vi "REWORK_MAIN.vi"() -> ()   [LabVIEW 2019]
uses:
  REWORK/MAIN/REWORK_station.ctl
  REWORK/MAIN/REWORK_header_data_display.ctl
  REWORK/ini/typedef/REWORK_all_config_info.ctl
  REWORK/ini/typedef/REWORK_main_ini_file.ctl
  REWORK/queues/typedef/REWORK_queue_refnums.ctl
  REWORK/queues/typedef/REWORK_MAIN_queue_element.ctl
  REWORK/MAIN/REWORK_MAIN_sequence_state.ctl
  REWORK/queues/typedef/REWORK_SCANNER_queue_element.ctl
  REWORK/SCANNER/REWORK_SCANNER_sequence_state.ctl
  REWORK/FGV/error_buffer/FGV_REWORK_error_buffer.ctl
  REWORK/TCP/REWORK_TCP_sequence_state.ctl
  REWORK/FGV/connection_reference/FGV_REWORK_connection_reference.ctl
  REWORK/FGV/DIAGNOSTICS_records_display/FGV_REWORK_DIAGNOSTICS_records_display.ctl
  REWORK/FGV/connection_indicators/FGV_REWORK_connection_indicators.ctl
  REWORK/FGV/DIAGNOSTICS_message_history_buffer/FGV_REWORK_DIAGNOSTICS_message_history_buffer.ctl
  REWORK/FGV/SQL_connection/FGV_REWORK_SQL_connection.ctl
  REWORK/FGV/login/FGV_REWORK_login.ctl
  REWORK/FGV/login/REWORK_login_refnums.ctl
  REWORK/FGV/REWORK_records_display/FGV_REWORK_records_display.ctl
  REWORK/FGV/REWORK_records_display/REWORK_references.ctl
  REWORK/FGV/REWORK_status_display/FGV_REWORK_status_display.ctl
  REWORK/FGV/REWORK_destination_selector/FGV_REWORK_destination_selector.ctl
  _misc/PLC_connection_status.ctl
  REWORK/MAIN/REWORK_thread.ctl
  <vilib>/Utility/miscctls.llb/LVRowAndColumnTypeDef.ctl
  _misc/AULocalize/SubVIs/RegisterVI.vi
  _misc/byte_array_parser/to_string.vi
  <vilib>/Instr/_visa.llb/VISA Configure Serial Port (Instr).vi
panel:
  out "app_title":string caption="A603 - Rework"
  in  "REWORK_toggle_all_results":bool
  in  "USER_login_logout":bool
  out "SQL_connections_indicator_global":bool=TRUE caption="SQL Connection Status:"
  out "PLC_connections_indicator_global":bool=TRUE caption="PLC Connection Status:"
  in  "STOP":bool
  out "ERROR_indicator_global":bool caption="Application Status:"
  out "current_access_level":i32=10 caption="Access level:"
  out "current_username":string="jlonga" caption="Logged in as:"
  in  "main_tab":enum32{"Rework", "Diagnostics", "Errors"}(tab)
  out "input_header":string caption="INPUT"
  in  "REWORK_clear_gear_data":bool
  in  "REWORK_read_data":bool
  in  "REWORK_destination":u16(ring) caption="Rework:" items=["NO REWORK POSSIBLE FOR THIS GEAR"]
  in  "REWORK_toggle_all_results":bool
  in  "REWORK_commit":bool
  in  "REWORK_records":i32(listbox)=-1
  out "REWORK_status":string
  in  "REWORK_gear_serial":string caption="Gear Serial:"
  in  "REWORK_station_filter":T1 caption="Station:" items=["ALL"=0, "Station 10"=10, "Station 20"=20, "Station 30"=30, "Station 40"=40, "Station 50"=50, "Station 60"=60, "Station 70"=70, "Station 80"=80, "Station 90"=90, "Station 100"=100, "Station 110"=110, "Station 120"=120, "Station 160"=165]
  out "REWORK_header_data_display":T2
  out "gear_info_summary_header":string caption="GEAR INFO SUMMARY"
  out "gear_serial_display":string
  in  "DIAGNOSTICS_save_log":bool
  in  "DIAGNOSTICS_show_messages":bool
  in  "DIAGNOSTICS_records":i32(listbox)
  in  "ERROR_records":i32(listbox)
  in  "ERROR_clear":bool
  out "ERROR_indicator_tab":bool
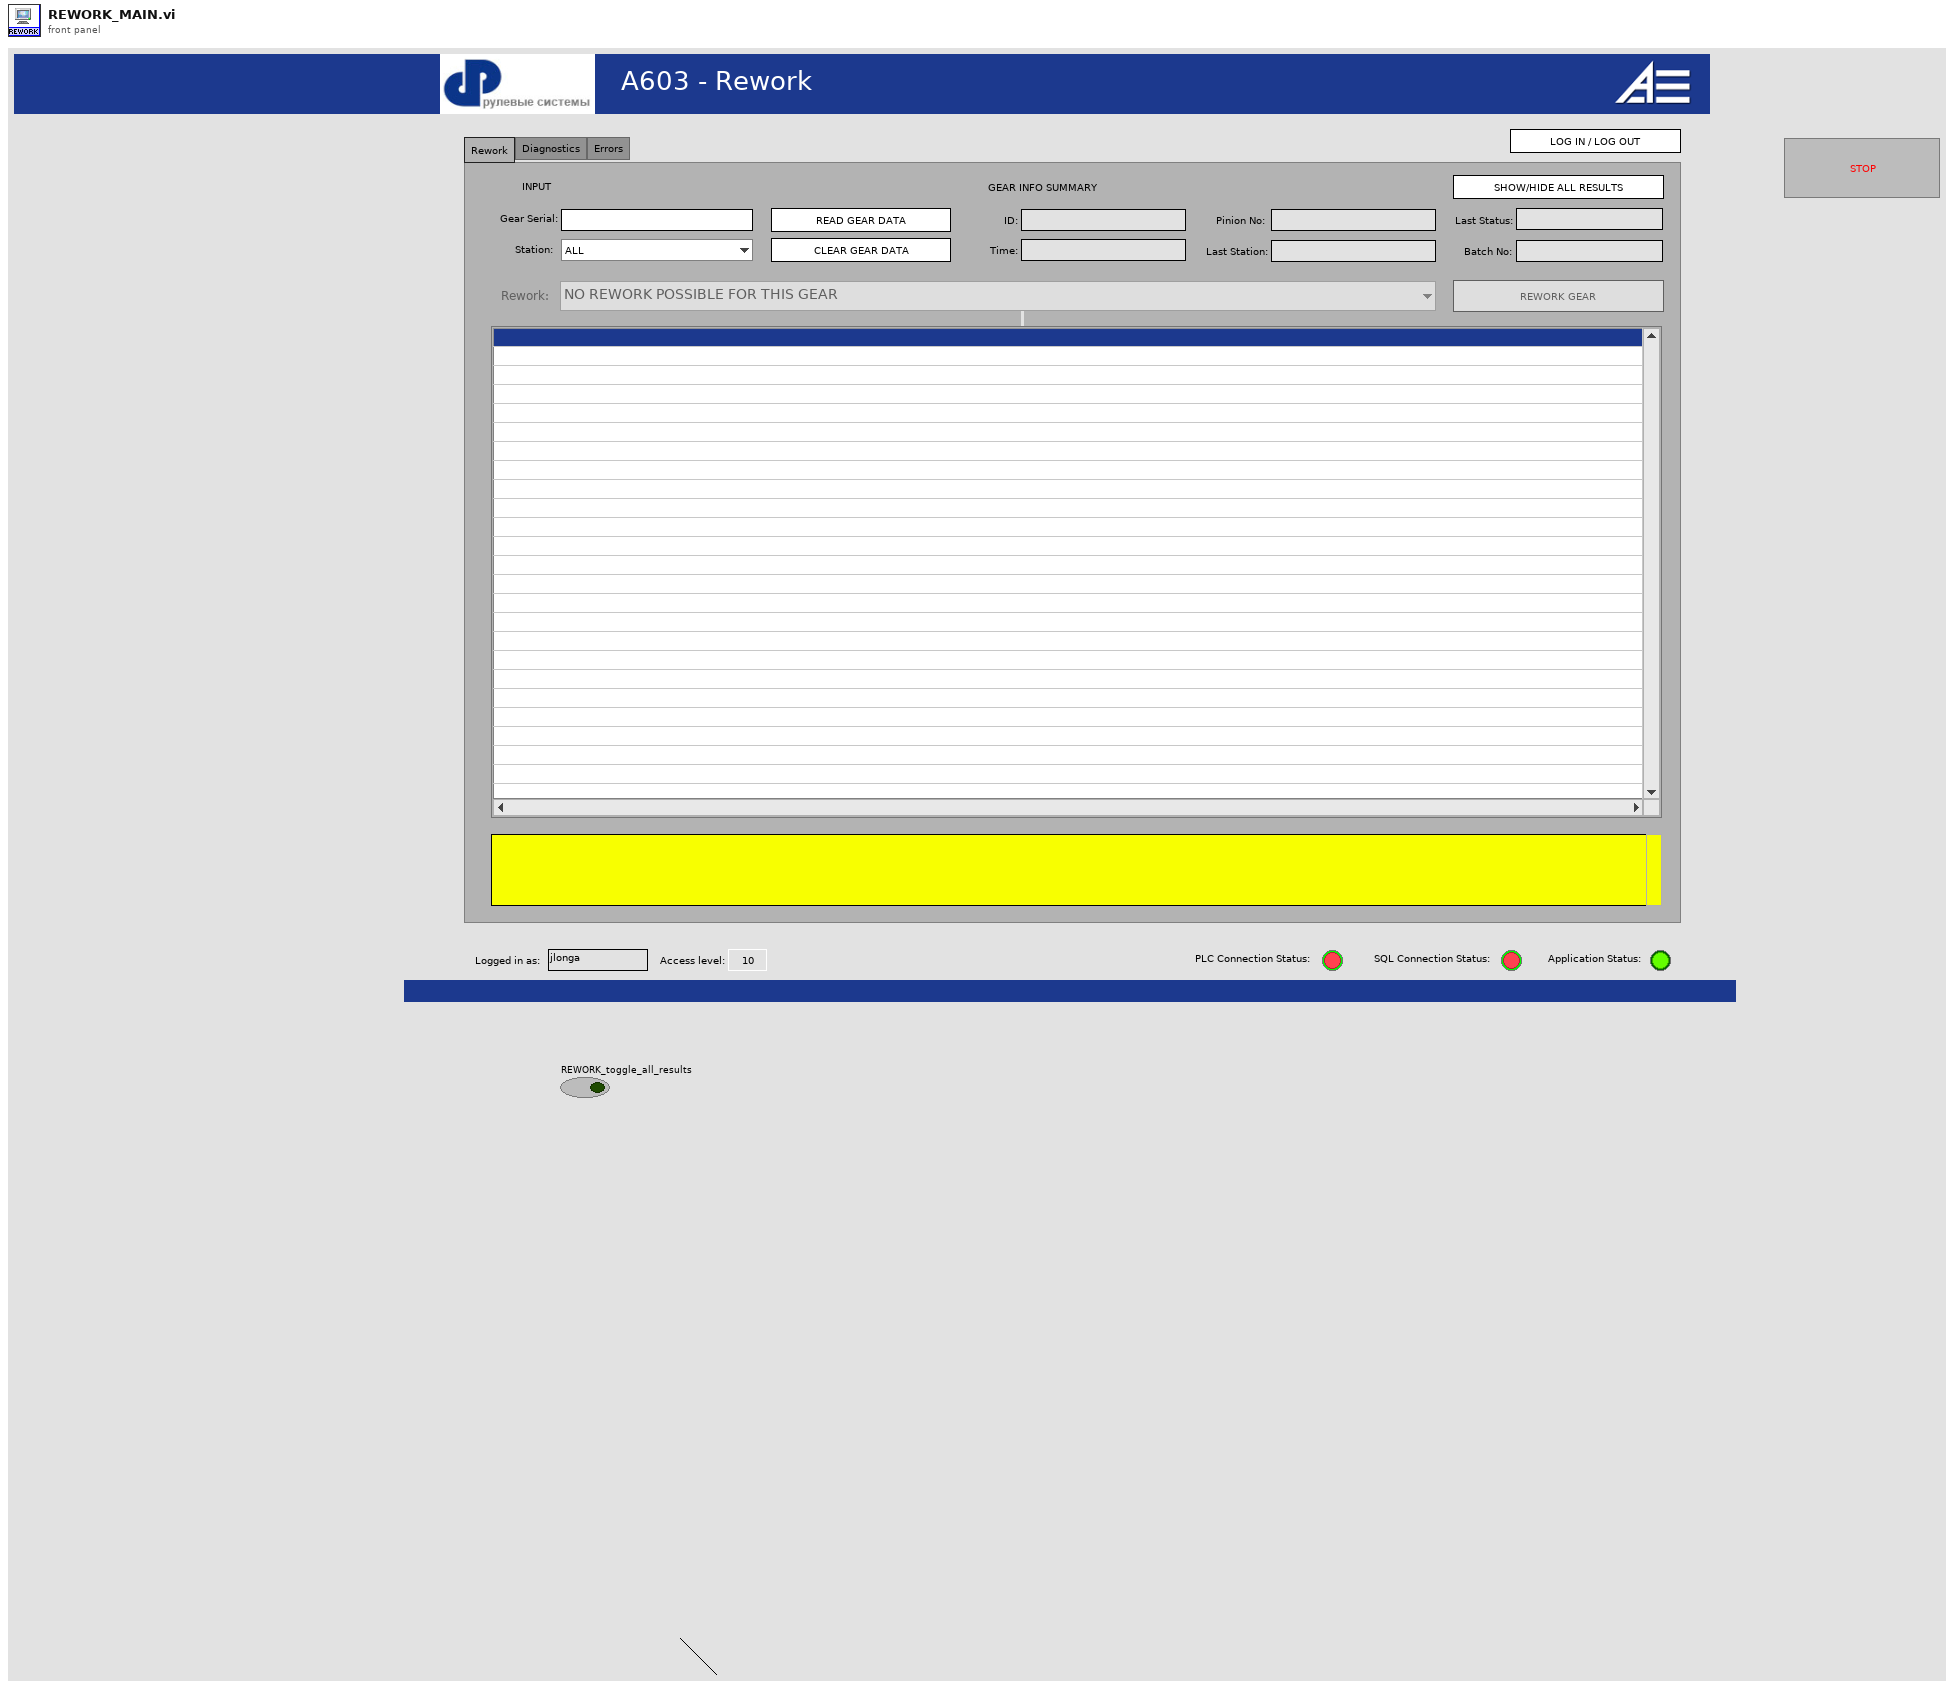
[diagram p1: front panel]
types:
  T1 = typedef "REWORK_station.ctl" = u16
  T2 = typedef "REWORK_header_data_display.ctl" = cluster{"ID":string, "creation_time":string, "last_station":string, "last_status":string, "pinion_serial":string, "batch_code":string}
  T3 = typedef "FGV_REWORK_destination_selector.ctl" = enum16{"initialize", "set_values", "display_values", "set_new_login", "enable", "disable", "disable_gray", "get_rework_to", "clear"}
  T4 = typedef "FGV_REWORK_status_display.ctl" = enum16{"initialize", "display", "clear"}
  T5 = typedef "REWORK_references.ctl" = cluster{"front_panel_reference":refnum<vi>, "SQL_listbox_reference":refnum<vi>, "REWORK_header_data_display":refnum<vi>}
  T6 = typedef "FGV_REWORK_records_display.ctl" = enum16{"initialize", "set_serial", "set_header", "set_operations", "set_results", "set_batches", "get_serial", "get_part_ID", "get_operation_IDs", "toggle_results", "show_all_results", "hide_all_results", "display", "clear"}
  T7 = typedef "REWORK_login_refnums.ctl" = cluster{"current_username":refnum<vi>, "current_access_level":refnum<vi>}
  T8 = typedef "FGV_REWORK_login.ctl" = enum16{"initialize", "login", "logout", "get_login_info"}
  T9 = typedef "REWORK_MAIN_sequence_state.ctl" = enum16{"initialize", "get_next_state", "parse_TCP", "send_TCP_response", "REWORK_commit", "USER_login", "USER_logout", "clear_gear_data", "error", "stop"}
  T10 = typedef "FGV_REWORK_SQL_connection.ctl" = enum16{"initialize", "connect", "read_tables", "read_columns", "SELECT", "INSERT", "UPDATE", "DELETE", "EXEC + headers", "EXEC", "TRANSACTION", "connection_active?", "disconnect"}
  T11 = typedef "FGV_REWORK_DIAGNOSTICS_message_history_buffer.ctl" = enum16{"initialize", "add_TCP_PLC_to_PC", "add_TCP_PC_to_PLC", "add_SQL_PC_to_DB", "add_SQL_transaction", "add_SQL_DB_to_PC", "get_all", "clear_all", "save_log"}
  T12 = typedef "FGV_REWORK_connection_indicators.ctl" = enum16{"initialize", "SQL_conn_ind_update", "PLC_conn_ind_update"}
  T13 = typedef "FGV_REWORK_DIAGNOSTICS_records_display.ctl" = enum16{"initialize", "set_PLC_IP", "set_PLC_Port", "set_PLC_connection_status", "set_SQL_connection_status", "get_all_info"}
  T14 = typedef "FGV_REWORK_connection_reference.ctl" = enum16{"initialize", "set_listener_ID", "set_connection_ID", "get", "KILL_ALL_CONNECTIONS", "killed?"}
  T15 = typedef "REWORK_TCP_sequence_state.ctl" = enum16{"initialize", "wait_for_connection", "handle_message", "error", "stop"}
  T16 = typedef "FGV_REWORK_error_buffer.ctl" = enum16{"initialize", "clear", "display", "get_status"}
  T17 = typedef "REWORK_SCANNER_sequence_state.ctl" = enum16{"initialize", "get_next_state", "read", "cancel_read", "error", "stop"}
  T18 = typedef "REWORK_all_config_info.ctl" = cluster{"main_ini_file":T19, "SQL Password":string, "queue_refnums":T20}
  T19 = typedef "REWORK_main_ini_file.ctl" = cluster{"SQL Driver":string, "SQL Server":string, "SQL Database":string, "SQL UID":string, "User table":string, "default language":string, "SCANNER COM port":u16, "SCANNER Baud rate":u32, "SCANNER Data bits":u16, "SCANNER Pairity":enum16{"None", "Odd", "Even", "Mark", "Space"}, "SCANNER Stop bits":u16, "SCANNER Flow control":u16, "SCANNER Termination char":u8, "ST 140 name":string, "ST 140 listener IP":string, "ST 140 listener port":u16, "logout timeout [ms]":i32}
  T20 = typedef "REWORK_queue_refnums.ctl" = cluster{"MAIN_queue":refnum<queue>, "SCANNER_queue":refnum<queue>, "SCANNER_data":refnum<queue>}
  T21 = typedef "PLC_connection_status.ctl" = enum16{"Connected", "Waiting", "Error", "-"}
  T22 = typedef "REWORK_MAIN_queue_element.ctl" = cluster{"state":T9, "variable":variant}
  T23 = enum16{"Standard", "Buffered", "CRLF", "Immediate"}
  T24 = typedef "REWORK_thread.ctl" = enum16{"MAIN", "TCP", "SCANNER"}
  T25 = typedef "REWORK_SCANNER_queue_element.ctl" = cluster{"state":T17, "variable":variant}
  T26 = typedef "LVRowAndColumnTypeDef.ctl" = cluster{"Row":i32, "Column":i32}
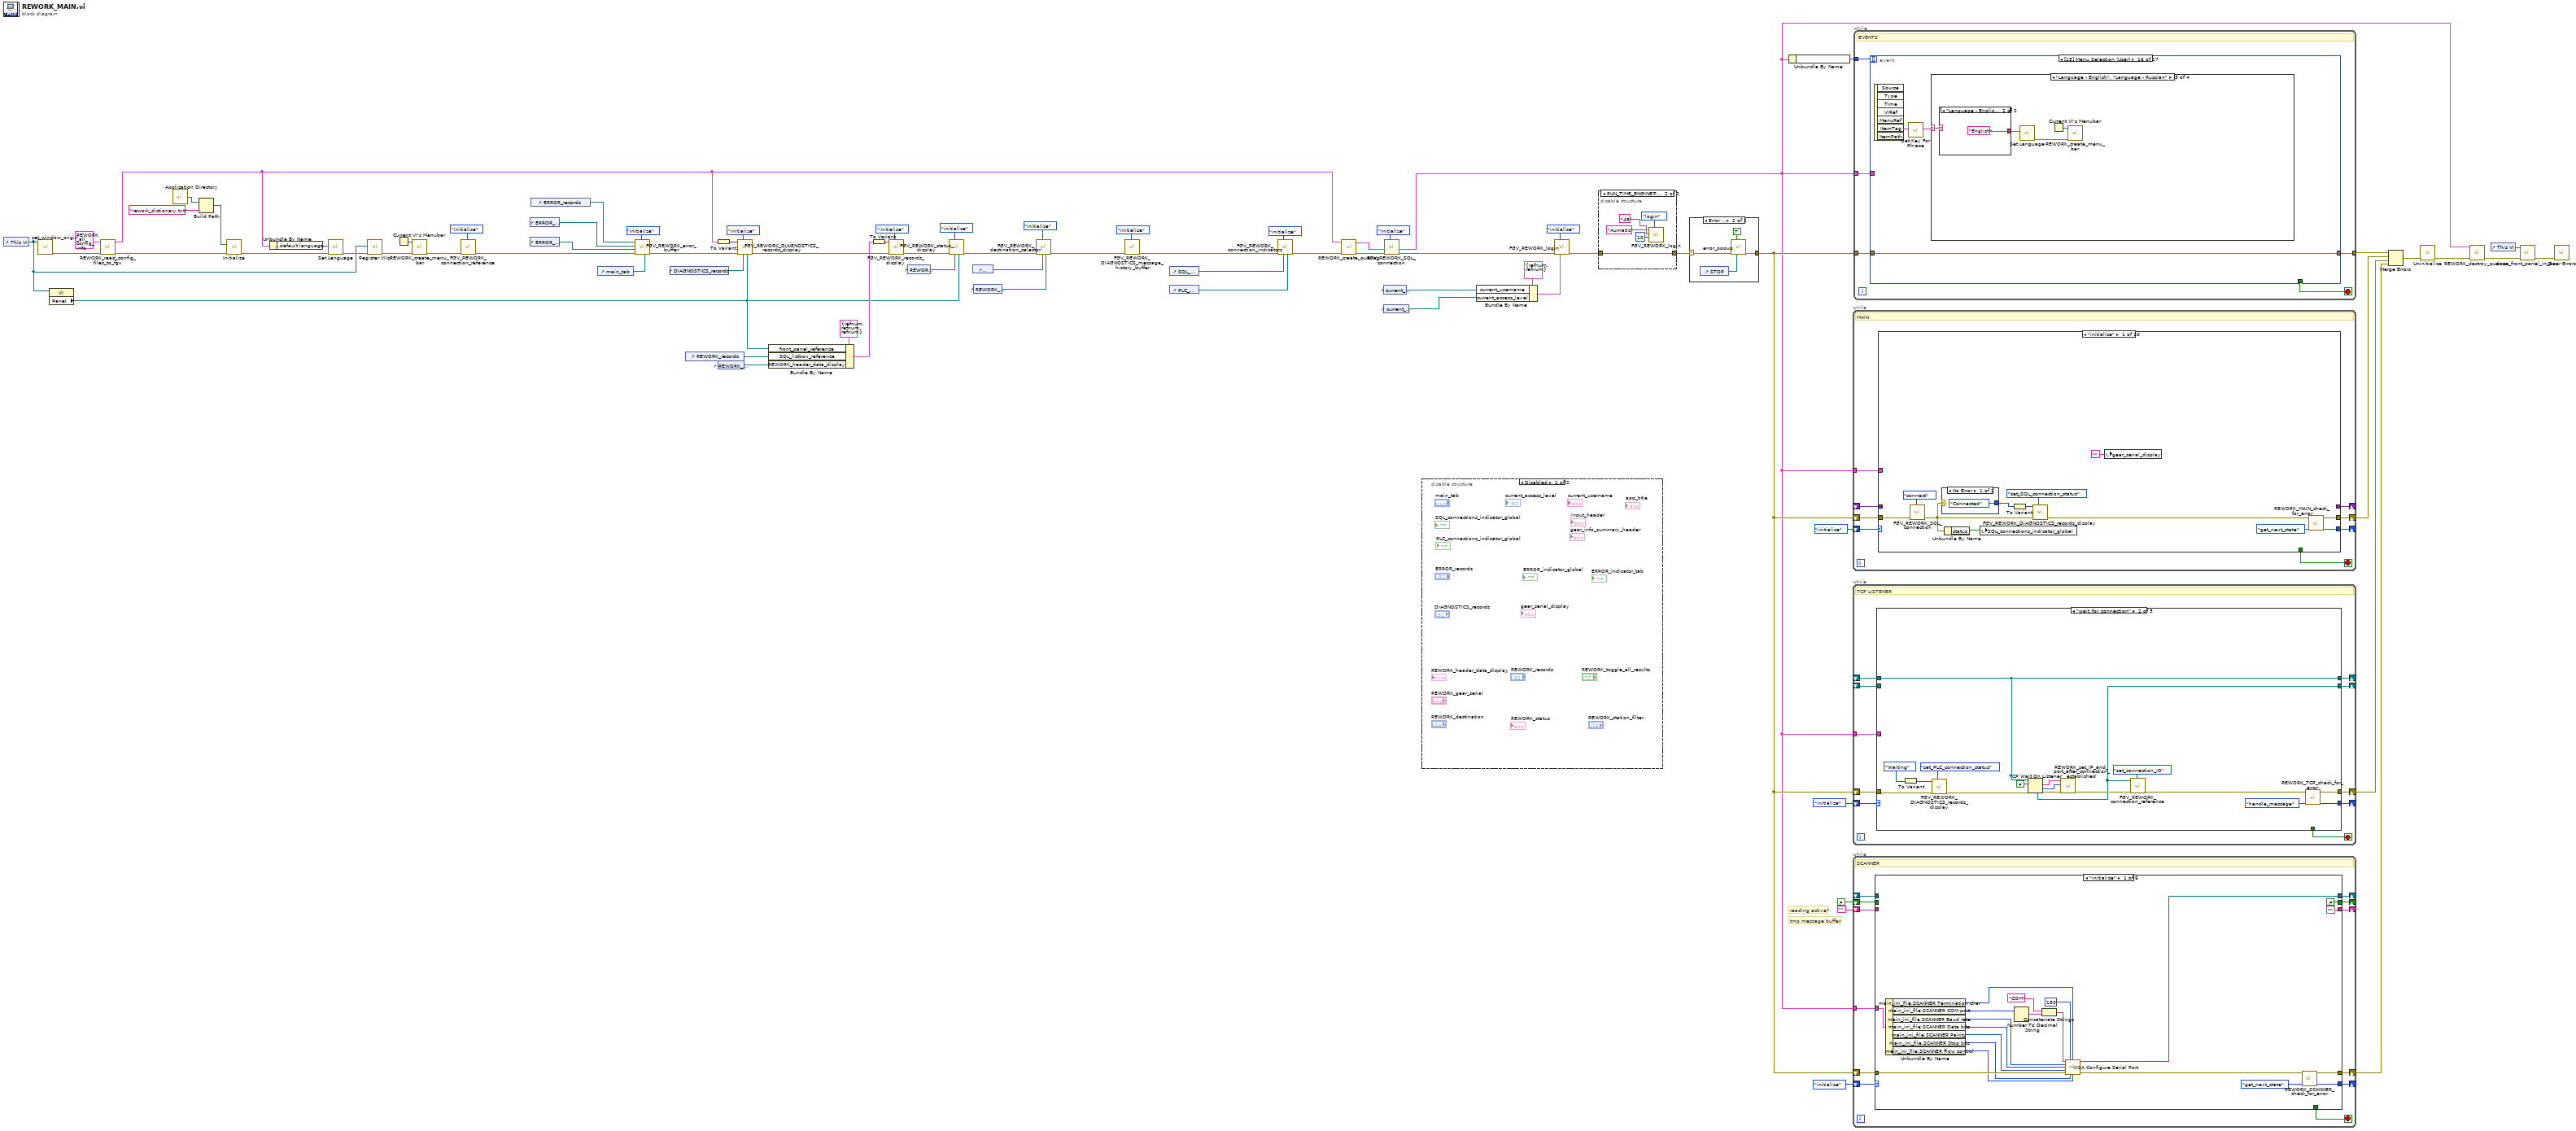
[diagram p0: block diagram]
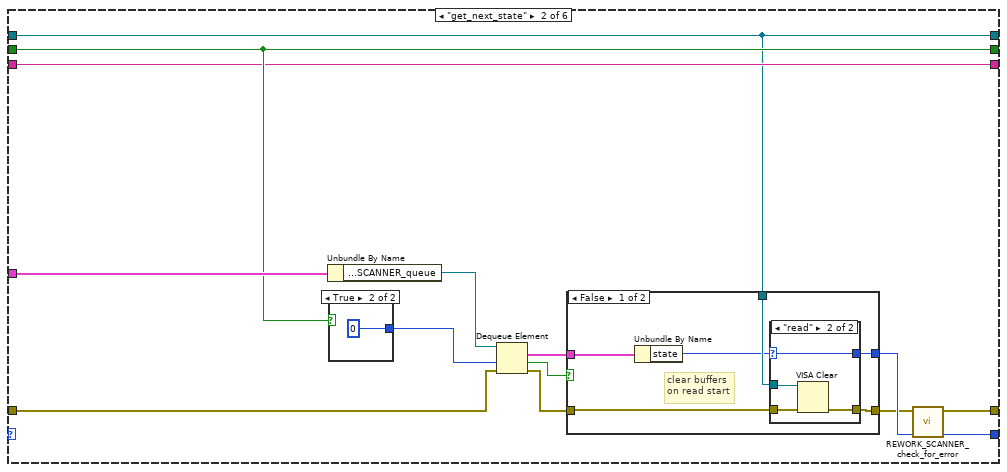
[diagram p4: hidden frame]
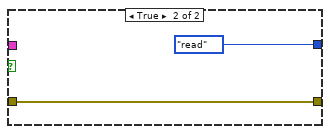
[diagram p6: hidden frame]
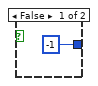
[diagram p7: hidden frame]
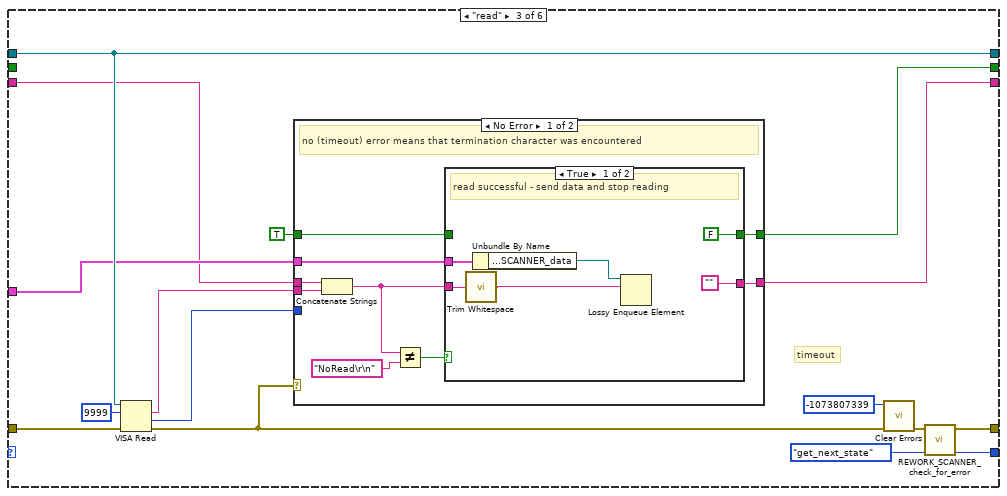
[diagram p8: hidden frame]
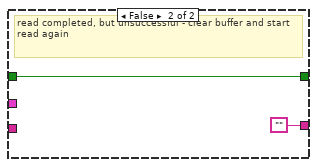
[diagram p9: hidden frame]
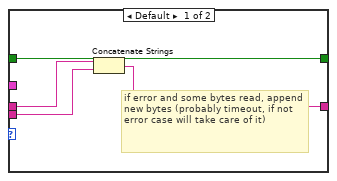
[diagram p11: hidden frame]
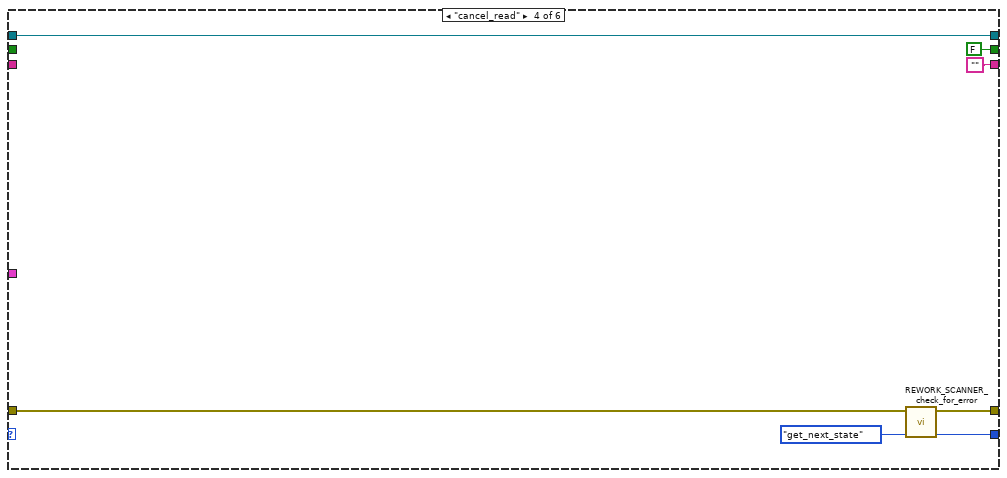
[diagram p12: hidden frame]
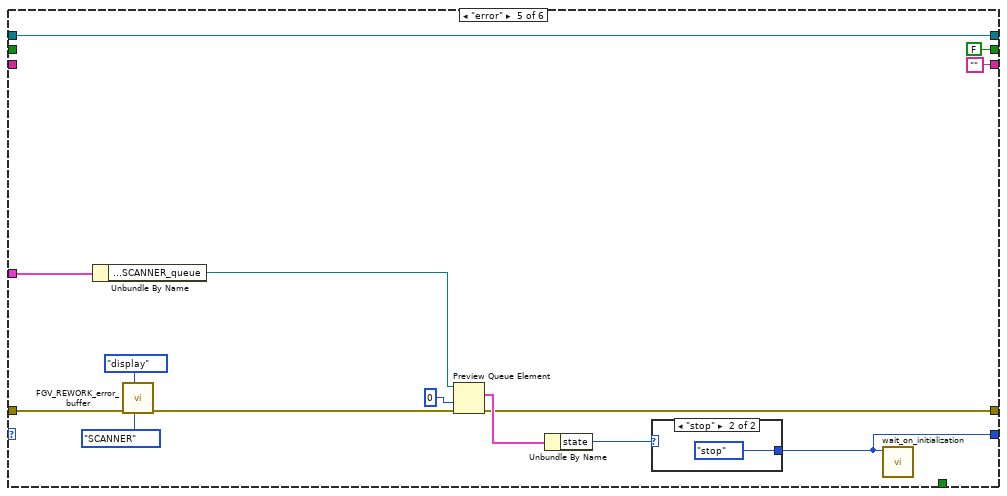
[diagram p13: hidden frame]
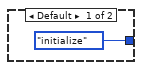
[diagram p14: hidden frame]
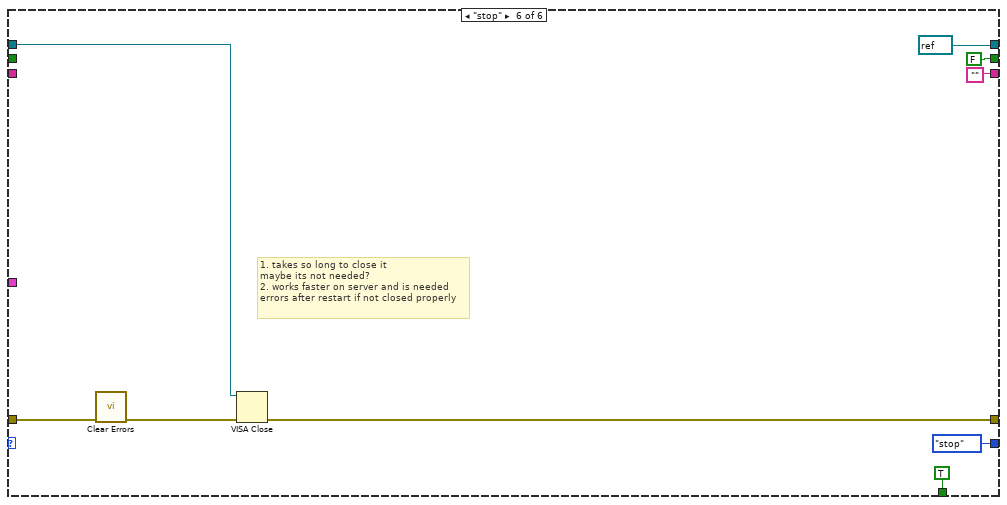
[diagram p15: hidden frame]
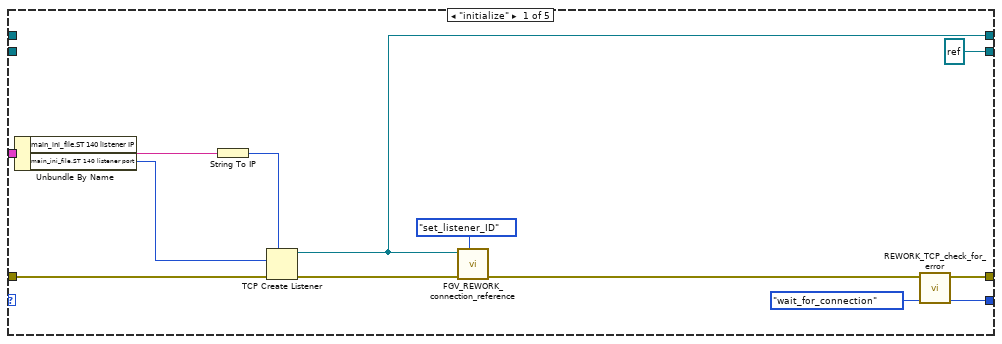
[diagram p16: hidden frame]
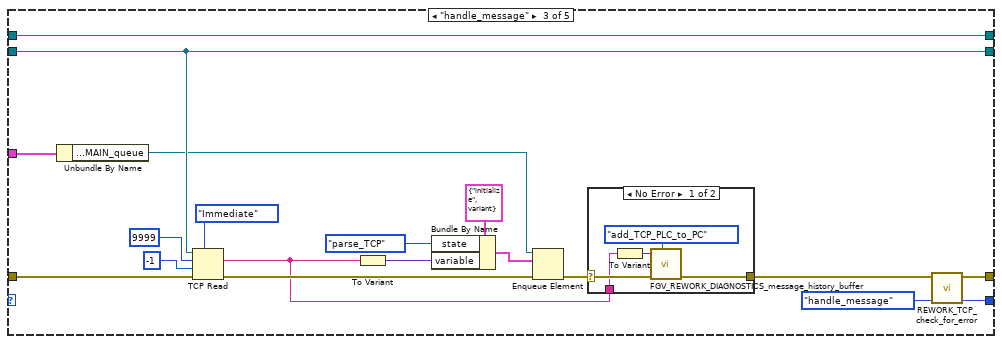
[diagram p17: hidden frame]
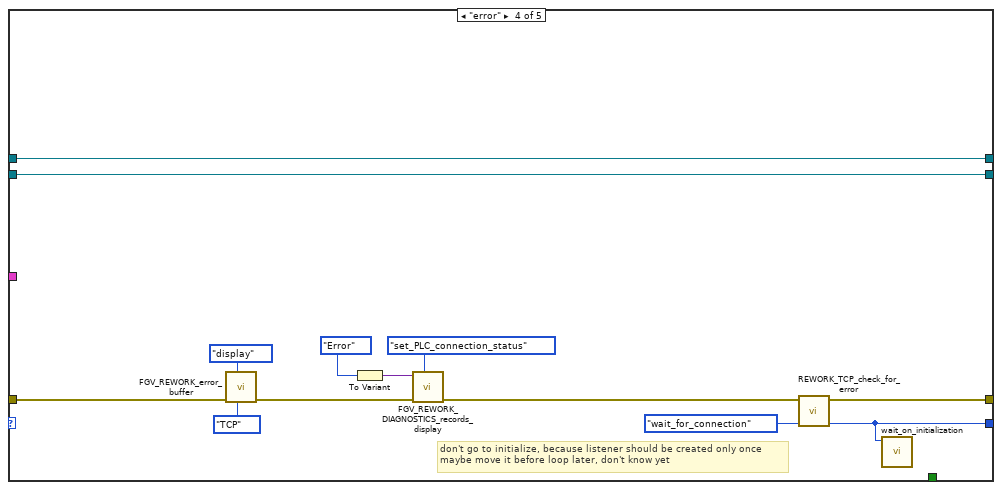
[diagram p19: hidden frame]
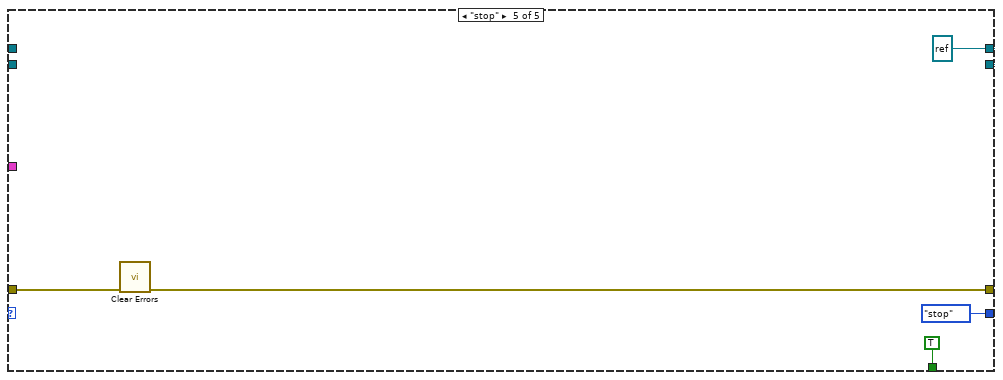
[diagram p20: hidden frame]
diagram:
  # "tmp message buffer"
  # "reading active?"
  n1 = control-ref of="This VI"() -> (w12:refnum<vi>)
  n2 = call "set_window_origin.vi"("this_vi_reference"=w12) -> ("error_out"=w4:errorcluster)  [unwired: 10 in]
  n3 = property class="VI"(reference=w12) -> ("Panel"=w28:refnum<vi>)  [unwired: 1 in, 2 out]
  n4 = call "REWORK_read_config_files_to_fgv.vi"("error_in"=w4, "all_config_info_in"=T18 {"main_ini_file"={"SQL Driver"="", "SQL Server"="", "SQL Database"="", "SQL UID"="", "User table"="", "default language"="", "SCANNER COM port"=0, "SCANNER Baud rate"=0, "SCANNER Data bits"=0, "SCANNER Pairity"=enum."None", "SCANNER Stop bits"=10, "SCANNER Flow control"=0, "SCANNER Termination char"=0, "ST 140 name"="", "ST 140 listener IP"="", "ST 140 listener port"=0, "logout timeout [ms]"=0}, "SQL Password"="", "queue_refnums"={"MAIN_queue"=refnum, "SCANNER_queue"=refnum, "SCANNER_data"=refnum}} ("all_config_info")) -> ("error_out"=w3:errorcluster, "all_config_info_out"=w2:T18)  [unwired: 8 in]
  n5 = call <vilib>:"Application Directory.vi"() -> ("Application Directory"=w15:path)
  n6 = Build Path(base path=w15, name or relative path="rework_dictionary.txt") -> (appended path=w13:path)
  n7 = call "Initialize.vi"("Dictionary File Path"=w13, "error in"=w3) -> ("error out"=w8:errorcluster)  [unwired: 8 in, 5 out]
  n8 = Unbundle By Name(w2) -> ("main_ini_file.default language"=w1:string)
  n9 = call "Set Language.vi"("error in"=w8, "Target Language (current lang)"=w1) -> ("error out"=w7:errorcluster)  [unwired: 8 in, 1 out]
  n10 = call-poly "Register VI(s).vi"("error in"=w7, "VI Ref"=w12) -> ("error out"=w6:errorcluster)  [unwired: 8 in, 1 out]
  n11 = Current VI's Menubar() -> (w9:refnum<k9>)
  n12 = call "REWORK_create_menu_bar.vi"("error_in"=w6, "menu_bar_refnum"=w9) -> ("error_out"=w5:errorcluster)  [unwired: 9 in]
  n13 = call "FGV_REWORK_connection_reference.vi"("options"=FGV_REWORK_connection_reference."initialize", "error_in"=w5) -> ("error_out"=w61:errorcluster)  [unwired: 6 in, 3 out]
  n14 = control-ref of="ERROR_indicator_tab"() -> (w64:refnum<vi>)
  n15 = control-ref of="ERROR_indicator_global"() -> (w65:refnum<vi>)
  n16 = control-ref of="ERROR_records"() -> (w63:refnum<vi>)
  n17 = control-ref of="main_tab"() -> (w66:refnum<vi>)
  n18 = call "FGV_REWORK_error_buffer.vi"("main_tab"=w66, "option"=FGV_REWORK_error_buffer."initialize", "error_in"=w61, "error_indicator_global"=w65, "error_indicator_tab"=w64, "error_display_ref"=w63) -> ("error_out"=w59:errorcluster)  [unwired: 4 in, 1 out]
  n19 = control-ref of="DIAGNOSTICS_records"() -> (w56:refnum<vi>)
  n20 = control-ref of="REWORK_records"() -> (w31:refnum<vi>)
  n21 = To Variant(anything=w2) -> (Variant=w57:variant)
  n22 = control-ref of="REWORK_header_data_display"() -> (w18:refnum<vi>)
  n23 = call "FGV_REWORK_DIAGNOSTICS_records_display.vi"("front_panel_reference"=w28, "SQL_listbox_reference"=w56, "options"=FGV_REWORK_DIAGNOSTICS_records_display."initialize", "error_in"=w59, "input"=w57) -> ("error_out"=w36:errorcluster)  [unwired: 5 in, 1 out]
  n24 = Bundle By Name(cluster=T5 {"front_panel_reference"=refnum, "SQL_listbox_reference"=refnum, "REWORK_header_data_display"=refnum} ("REPORTS_references"), "front_panel_reference"=w28, "SQL_listbox_reference"=w31, "REWORK_header_data_display"=w18) -> (w32:T5)
  n25 = To Variant(anything=w32) -> (Variant=w33:variant)
  n26 = call "FGV_REWORK_records_display.vi"("options"=FGV_REWORK_records_display."initialize", "error_in"=w36, "input"=w33) -> ("error_out"=w30:errorcluster)  [unwired: 7 in, 1 out]
  n27 = control-ref of="REWORK_status"() -> (w27:refnum<vi>)
  n28 = call "FGV_REWORK_status_display.vi"("front_panel_reference"=w28, "REP_status_display_reference"=w27, "options"=FGV_REWORK_status_display."initialize", "error_in"=w30) -> ("error_out"=w26:errorcluster)  [unwired: 7 in]
  n29 = control-ref of="REWORK_destination"() -> (w23:refnum<vi>)
  n30 = control-ref of="REWORK_commit"() -> (w21:refnum<vi>)
  n31 = call "FGV_REWORK_destination_selector.vi"("REWORK_commit"=w21, "REWORK_destination"=w23, "options"=FGV_REWORK_destination_selector."initialize", "error_in"=w26) -> ("error_out"=w25:errorcluster)  [unwired: 6 in, 1 out]
  n32 = call "FGV_REWORK_DIAGNOSTICS_message_history_buffer.vi"("options"=FGV_REWORK_DIAGNOSTICS_message_history_buffer."initialize", "error_in"=w25) -> ("error_out"=w51:errorcluster)  [unwired: 8 in, 1 out]
  n33 = control-ref of="SQL_connections_indicator_global"() -> (w53:refnum<vi>)
  n34 = control-ref of="PLC_connections_indicator_global"() -> (w52:refnum<vi>)
  n35 = call "FGV_REWORK_connection_indicators.vi"("PLC_connections_indicator_global"=w52, "SQL_connections_indicator_global"=w53, "options"=FGV_REWORK_connection_indicators."initialize", "error_in"=w51) -> ("error_out"=w55:errorcluster)  [unwired: 7 in]
  n36 = call "REWORK_create_queues.vi"("error_in"=w55, "all_config_info_in"=w2) -> ("error_out"=w45:errorcluster, "all_config_info_out"=w44:T18)  [unwired: 8 in]
  n37 = control-ref of="current_username"() -> (w39:refnum<vi>)
  n38 = control-ref of="current_access_level"() -> (w38:refnum<vi>)
  n39 = call "FGV_REWORK_SQL_connection.vi"("options"=FGV_REWORK_SQL_connection."initialize", "error_in"=w45, "all_config_info_in"=w44) -> ("error_out"=w22:errorcluster, "all_config_info_out"=w20:T18)  [unwired: 4 in, 3 out]
  n40 = disable-structure shown="Disabled" {
    frame Disabled {
    }
    frame Enabled {
    }
  }
  n41 = Bundle By Name(cluster=T7 {"current_username"=refnum, "current_access_level"=refnum} ("login_refnums"), "current_username"=w39, "current_access_level"=w38) -> (w37:T7)
  n42 = call "FGV_REWORK_login.vi"("login_refnums"=w37, "options"=FGV_REWORK_login."initialize", "error_in"=w22) -> ("error_out"=w17:errorcluster)  [unwired: 5 in, 3 out]
  n43 = disable-structure shown="RUN_TIME_ENGINE==False" {
    disable-tunnel: w17 -> [w76 w81]
    disable-tunnel: [w76 w81] -> w16
    frame condition #0 {
    }
    frame condition #1 (active) {
      n44 = call "FGV_REWORK_login.vi"("options"=FGV_REWORK_login."login", "access_level_in"=10, "username_in"="Aumatic", "ID_in"="45") -> ()  [unwired: 4 in, 4 out]
    }
  }
  n45 = case shown="Error .." w16 {
    selector: w16 -> [w82 w85]
    tunnel: [w82 w86] -> w71
    frame No Error {
    }
    frame Error {
      n46 = control-ref of="STOP"() -> (w84:refnum<vi>)
      n47 = call "error_popup.vi"("STOP_button_reference"=w84, "EXIT App If Error? (F)"=TRUE, "error_in"=w85) -> ("error_out"=w86:errorcluster)  [unwired: 8 in]
    }
  }
  n48 = Unbundle By Name(w20) -> ("main_ini_file.logout timeout [ms]"=w19:i32)
  n49 = while {
    tunnel: w20 -> [w89]
    shift-right: [w92] -> w48
    shift-left: w71 -> [w93]
    shift-right: [w91] -> _
    shift-left: REWORK_MAIN_sequence_state."initialize" ("SQL_EDITOR_sequence_state") -> [w94]
    shift-right: [w88] -> _
    shift-left: _ -> [w87]
    stop <- w90 stop-if-true
    # "MAIN"
    n50 = case shown="\"initialize\"" w94 {
      tunnel: w93 -> [w105 w113 w126 w203 w249 w259 w301 w309 w320 w347]
      tunnel: [w104 w117 w130 w213 w256 w278 w305 w316 w319 w347] -> w92
      tunnel: [w103 w116 w129 w212 w255 w277 w304 w315 w318 REWORK_MAIN_sequence_state."stop" ("ST_TCP_sequence_state")] -> w91
      tunnel: [_ _ _ _ _ _ _ _ _ TRUE] -> w90
      tunnel: w89 -> [_ w111 _ _ _ w258 _ _ w317 _]
      tunnel: [_ w110 w119 _ w225 _ _ _ _ _] -> w88
      tunnel: w87 -> [_ _ w125 w202 _ w257 _ _ _ _]
      frame "initialize" {
        n51 = call "FGV_REWORK_SQL_connection.vi"("options"=FGV_REWORK_SQL_connection."connect", "error_in"=w105) -> ("error_out"=w99:errorcluster)  [unwired: 5 in, 4 out]
        n52 = case shown="No Error" w99 {
          tunnel: [PLC_connection_status."Connected" PLC_connection_status."Error"] -> w97
          frame No Error {
          }
          frame Error {
          }
        }
        n53 = Unbundle By Name(w99) -> ("status"=w102:bool)
        n54 = local write "SQL_connections_indicator_global"(w102) -> ()
        n55 = To Variant(anything=w97) -> (Variant=w98:variant)
        n56 = call "FGV_REWORK_DIAGNOSTICS_records_display.vi"("options"=FGV_REWORK_DIAGNOSTICS_records_display."set_SQL_connection_status", "error_in"=w99, "input"=w98) -> ("error_out"=w100:errorcluster)  [unwired: 7 in, 1 out]
        n57 = local write "gear_serial_display"("") -> ()
        n58 = call "REWORK_MAIN_check_for_error.vi"("MAIN_loop_state_in"=REWORK_MAIN_sequence_state."get_next_state", "error_in"=w100) -> ("MAIN_loop_state_out"=w103:T9, "error_out"=w104:errorcluster)  [unwired: 8 in]
      }
      frame "get_next_state" {
        n59 = Unbundle By Name(w111) -> ("queue_refnums.MAIN_queue"=w114:refnum<queue>)
        n60 = Dequeue Element(queue=w114, error in (no error)=w113) -> (element=w115:T22, error out=w112:errorcluster)  [unwired: 1 in, 2 out]
        n61 = Unbundle By Name(w115) -> ("variable"=w110:variant, "state"=w109:T9)
        n62 = call "REWORK_MAIN_check_for_error.vi"("MAIN_loop_state_in"=w109, "error_in"=w112) -> ("MAIN_loop_state_out"=w116:T9, "error_out"=w117:errorcluster)  [unwired: 8 in]
      }
      frame "parse_TCP" {
        # "command number"
        n63 = Variant To Data(error in=w126, type="", Variant=w125) -> (data=w127:string, error out=w122:errorcluster)
        n64 = String To Byte Array(string=w127) -> (unsigned byte array=w120:u8[])
        n65 = Index Array(array=w120, index=0) -> (element=w123:u8)
        n66 = case shown="Default" w123 {
          selector: w123 -> [w138 _ w196]
          tunnel: w122 -> [w161 w190 _]
          tunnel: [w144 w173 w195] -> w121
          tunnel: w120 -> [w154 w183 _]
          tunnel: [w135 _ _] -> w119
          tunnel: [REWORK_MAIN_sequence_state."send_TCP_response" ("MAIN_loop_state_in") REWORK_MAIN_sequence_state."get_next_state" ("MAIN_loop_state_in") REWORK_MAIN_sequence_state."error" ("MAIN_loop_state_in")] -> w118
          frame 1 {
            # "after changes update command 101 also"
            n67 = call-poly "byte_array_parser.vi"("error_in"=w161, "string_length"=20, "variable_start_index"=3, "byte_array"=w154) -> ("error_out"=w159:errorcluster, "string"=w133:string)  [unwired: 6 in]
            n68 = To Variant(anything=w133) -> (Variant=w149:variant)
            n69 = Format Into String(format string="select top 1 PRODUCTION_PARTS.ID, PRODUCTION_PARTS.CREATION_TIME, PRODUCTION_PARTS.LAST_STATION_NMB, PRODUCTION_PARTS.LAST_STATUS, PRODUCTION_PINIONS.PINION_SERIAL, DOCK_AUDIT_BATCHES.BATCH_CODE, PRODUCTION_PARTS.PINION_ID, PRODUCTION_PARTS.BATCH_ID\nfrom PRODUCTION_PARTS \nleft join PRODUCTION_PINIONS on PRODUCTION_PARTS.PINION_ID = PRODUCTION_PINIONS.ID\nleft join DOCK_AUDIT_BATCHES on PRODUCTION_PARTS.BATCH_ID = DOCK_AUDIT_BATCHES.ID\nwhere PART_SERIAL = '%s'", w133) -> (resulting string=w157:string)  [unwired: 2 in, 1 out]
            n70 = local write "REWORK_gear_serial"(w133) -> ()
            n71 = call "FGV_REWORK_records_display.vi"("options"=FGV_REWORK_records_display."set_serial", "input"=w149) -> ()  [unwired: 8 in, 2 out]
            n72 = call "FGV_REWORK_SQL_connection.vi"("options"=FGV_REWORK_SQL_connection."SELECT", "error_in"=w159, "SQL_statement"=w157) -> ("error_out"=w156:errorcluster, "SQL_result"=w145:variant, "executed_SQL_statement"=w146:string)  [unwired: 4 in, 2 out]
            n73 = call "FGV_REWORK_records_display.vi"("options"=FGV_REWORK_records_display."set_header", "error_in"=w156, "input"=w145) -> ("error_out"=w148:errorcluster)  [unwired: 7 in, 1 out]
            n74 = local write "gear_serial_display"(w133) -> ()
            n75 = call "REWORK_get_operations_and_results.vi"("executed_SQL_statement_in"=w146, "error_in"=w148, "SQL_result"=w145) -> ("error_out"=w147:errorcluster, "executed_SQL_statement_out"=w142:string)  [unwired: 7 in]
            n76 = local read "REWORK_station_filter"() -> (w151:T1)
            n77 = To Variant(anything=w151) -> (Variant=w152:variant)
            n78 = call "FGV_REWORK_records_display.vi"("options"=FGV_REWORK_records_display."display", "error_in"=w147, "input"=w152) -> ("error_out"=w139:errorcluster)  [unwired: 7 in, 1 out]
            n79 = local write "REWORK_toggle_all_results"(FALSE ("REWORK_toggle_all_results")) -> ()
            n80 = call-poly "Get Localized Phrase Compact Interface.vi"("Key"="SHOW ALL RESULTS" ("Boolean Text.Text")) -> ("Translated Phrase"=w131:string)
            n81 = property on="REWORK_toggle_all_results" class="Bool"("BoolText.Text"=w131) -> ()  [unwired: 2 in, 2 out]
            n82 = Build Array(w138, u8 1 ("element")) -> (w136:u8[])
            n83 = call "FGV_REWORK_status_display.vi"("options"=FGV_REWORK_status_display."display", "error_in"=w139, "SQL_statement"=w142, "display_source"="READ GEAR DATA") -> ("error_out"=w144:errorcluster)  [unwired: 7 in]
            n84 = To Variant(anything=w136) -> (Variant=w135:variant)
          }
          frame 101 {
            n85 = call-poly "byte_array_parser.vi"("error_in"=w190, "string_length"=20, "variable_start_index"=3, "byte_array"=w183) -> ("error_out"=w188:errorcluster, "string"=w165:string)  [unwired: 6 in]
            n86 = To Variant(anything=w165) -> (Variant=w178:variant)
            n87 = Format Into String(format string="select top 1 PRODUCTION_PARTS.ID, PRODUCTION_PARTS.CREATION_TIME, PRODUCTION_PARTS.LAST_STATION_NMB, PRODUCTION_PARTS.LAST_STATUS, PRODUCTION_PINIONS.PINION_SERIAL, DOCK_AUDIT_BATCHES.BATCH_CODE, PRODUCTION_PARTS.PINION_ID, PRODUCTION_PARTS.BATCH_ID\nfrom PRODUCTION_PARTS \nleft join PRODUCTION_PINIONS on PRODUCTION_PARTS.PINION_ID = PRODUCTION_PINIONS.ID\nleft join DOCK_AUDIT_BATCHES on PRODUCTION_PARTS.BATCH_ID = DOCK_AUDIT_BATCHES.ID\nwhere PART_SERIAL = '%s'", w165) -> (resulting string=w186:string)  [unwired: 2 in, 1 out]
            n88 = local write "REWORK_gear_serial"(w165) -> ()
            n89 = call "FGV_REWORK_records_display.vi"("options"=FGV_REWORK_records_display."set_serial", "input"=w178) -> ()  [unwired: 8 in, 2 out]
            n90 = call "FGV_REWORK_SQL_connection.vi"("options"=FGV_REWORK_SQL_connection."SELECT", "error_in"=w188, "SQL_statement"=w186) -> ("error_out"=w185:errorcluster, "SQL_result"=w174:variant, "executed_SQL_statement"=w175:string)  [unwired: 4 in, 2 out]
            n91 = call "FGV_REWORK_records_display.vi"("options"=FGV_REWORK_records_display."set_header", "error_in"=w185, "input"=w174) -> ("error_out"=w177:errorcluster)  [unwired: 7 in, 1 out]
            n92 = local write "gear_serial_display"(w165) -> ()
            n93 = call "REWORK_get_operations_and_results.vi"("executed_SQL_statement_in"=w175, "error_in"=w177, "SQL_result"=w174) -> ("error_out"=w176:errorcluster, "executed_SQL_statement_out"=w171:string)  [unwired: 7 in]
            n94 = local read "REWORK_station_filter"() -> (w180:T1)
            n95 = To Variant(anything=w180) -> (Variant=w181:variant)
            n96 = call "FGV_REWORK_records_display.vi"("options"=FGV_REWORK_records_display."display", "error_in"=w176, "input"=w181) -> ("error_out"=w167:errorcluster)  [unwired: 7 in, 1 out]
            n97 = local write "REWORK_toggle_all_results"(FALSE ("REWORK_toggle_all_results")) -> ()
            n98 = call-poly "Get Localized Phrase Compact Interface.vi"("Key"="SHOW ALL RESULTS" ("Boolean Text.Text")) -> ("Translated Phrase"=w164:string)
            n99 = property on="REWORK_toggle_all_results" class="Bool"("BoolText.Text"=w164) -> ()  [unwired: 2 in, 2 out]
            n100 = call "FGV_REWORK_status_display.vi"("options"=FGV_REWORK_status_display."display", "error_in"=w167, "SQL_statement"=w171, "display_source"="READ GEAR DATA") -> ("error_out"=w173:errorcluster)  [unwired: 7 in]
          }
          frame Default {
            n101 = call-poly "Get Localized Phrase Compact Interface.vi"("Key"="Unknown command from PLC received. Command: %d" ("source")) -> ("Translated Phrase"=w193:string)
            n102 = Format Into String(format string=w193, w196) -> (resulting string=w199:string)  [unwired: 2 in, 1 out]
            n103 = Bundle By Name(cluster=errorcluster {"status"=TRUE, "code"=500, "source"=""} ("error_out"), "source"=w199) -> (w195:errorcluster)
          }
        }
        n104 = call "REWORK_MAIN_check_for_error.vi"("MAIN_loop_state_in"=w118, "error_in"=w121) -> ("MAIN_loop_state_out"=w129:T9, "error_out"=w130:errorcluster)  [unwired: 8 in]
      }
      frame "send_TCP_response" {
        n105 = Variant To Data(error in=w203, type=u8[] [], Variant=w202) -> (data=w206:u8[], error out=w205:errorcluster)
        n106 = call "FGV_REWORK_connection_reference.vi"("options"=FGV_REWORK_connection_reference."get", "error_in"=w205) -> ("error_out"=w210:errorcluster, "connection_ID_out"=w209:refnum<k5>)  [unwired: 6 in, 2 out]
        n107 = TCP Write(connection ID=w209, data in=w206, error in (no error)=w210) -> (error out=w207:errorcluster)  [unwired: 1 in, 2 out]
        n108 = Byte Array To String(unsigned byte array=w206) -> (string=w204:string)
        n109 = case shown="No Error" w207 {
          selector: w207 -> [w218 w219]
          tunnel: [w217 w219] -> w201
          tunnel: w204 -> [w216 _]
          frame No Error {
            n110 = To Variant(anything=w216) -> (Variant=w215:variant)
            n111 = call "FGV_REWORK_DIAGNOSTICS_message_history_buffer.vi"("options"=FGV_REWORK_DIAGNOSTICS_message_history_buffer."add_TCP_PC_to_PLC", "error_in"=w218, "input"=w215) -> ("error_out"=w217:errorcluster)  [unwired: 7 in, 1 out]
          }
          frame Error {
          }
        }
        n112 = call "REWORK_MAIN_check_for_error.vi"("MAIN_loop_state_in"=REWORK_MAIN_sequence_state."get_next_state", "error_in"=w201) -> ("MAIN_loop_state_out"=w212:T9, "error_out"=w213:errorcluster)  [unwired: 8 in]
      }
      frame "REWORK_commit" {
        # "to refresh rework data"
        n113 = call "FGV_REWORK_records_display.vi"("options"=FGV_REWORK_records_display."get_part_ID", "error_in"=w249) -> ("error_out"=w248:errorcluster, "output"=w245:variant)  [unwired: 8 in]
        n114 = call "FGV_REWORK_login.vi"("options"=FGV_REWORK_login."get_login_info", "error_in"=w248) -> ("error_out"=w243:errorcluster, "ID_out"=w250:string)  [unwired: 6 in, 2 out]
        n115 = Variant To Data(type="", Variant=w245) -> (data=w244:string)  [unwired: 1 in, 1 out]
        n116 = local read "REWORK_destination"() -> (w237:u16)
        n117 = To Variant(anything=w237) -> (Variant=w238:variant)
        n118 = call "FGV_REWORK_destination_selector.vi"("options"=FGV_REWORK_destination_selector."get_rework_to", "error_in"=w243, "input"=w238) -> ("error_out"=w242:errorcluster, "output"=w239:variant)  [unwired: 7 in]
        n119 = Variant To Data(type="", Variant=w239) -> (data=w223:string)  [unwired: 1 in, 1 out]
        n120 = Format Into String(format string="EXEC PerformRework @PartID = %s, @UserID = %s, @ReworkTo = %s", w244, w250, w223) -> (resulting string=w224:string)  [unwired: 2 in, 1 out]
        n121 = call "FGV_REWORK_SQL_connection.vi"("options"=FGV_REWORK_SQL_connection."EXEC", "error_in"=w242, "SQL_statement"=w224) -> ("error_out"=w222:errorcluster, "SQL_result"=w220:variant, "executed_SQL_statement"=w233:string)  [unwired: 4 in, 2 out]
        n122 = call "FGV_REWORK_records_display.vi"("options"=FGV_REWORK_records_display."get_serial") -> ("output"=w228:variant)  [unwired: 9 in, 1 out]
        n123 = call "REWORK_parse_rework_commit_response.vi"("error_in"=w222, "sql_results_in"=w220) -> ("error_out"=w221:errorcluster)  [unwired: 9 in]
        n124 = Variant To Data(type="", Variant=w228) -> (data=w227:string)  [unwired: 1 in, 1 out]
        n125 = Byte Array To String(unsigned byte array=u8[] [1, 255, 255]) -> (string=w232:string)
        n126 = call "FGV_REWORK_status_display.vi"("options"=FGV_REWORK_status_display."display", "error_in"=w221, "SQL_statement"=w233, "display_source"="REWORK") -> ("error_out"=w234:errorcluster)  [unwired: 7 in]
        n127 = Concatenate Strings(w232, w227) -> (w226:string)
        n128 = To Variant(anything=w226) -> (Variant=w225:variant)
        n129 = call "REWORK_MAIN_check_for_error.vi"("MAIN_loop_state_in"=REWORK_MAIN_sequence_state."parse_TCP", "error_in"=w234) -> ("MAIN_loop_state_out"=w255:T9, "error_out"=w256:errorcluster)  [unwired: 8 in]
      }
      frame "USER_login" {
        n130 = Variant To Data(error in=w259, type="", Variant=w257) -> (data=w274:string, error out=w265:errorcluster)
        n131 = Unbundle By Name(w258) -> ("main_ini_file.User table"=w269:string)
        n132 = call "Hash String with SHA-256.vi"("error_n"=w265, "string"=w274) -> ("error_out"=w268:errorcluster, "hash"=w275:string)  [unwired: 8 in]
        n133 = Format Into String(format string="select ID, USER_NAME, PROXY_APP\nfrom %s\nwhere BARCODE_HASH = '%s'\norder by ID desc", w269, w275) -> (resulting string=w266:string)  [unwired: 2 in, 1 out]
        n134 = call "FGV_REWORK_SQL_connection.vi"("options"=FGV_REWORK_SQL_connection."SELECT", "error_in"=w268, "SQL_statement"=w266) -> ("error_out"=w267:errorcluster, "SQL_result"=w270:variant)  [unwired: 4 in, 3 out]
        n135 = Variant To Data(error in=w267, type=string[][] [], Variant=w270) -> (data=w272:string[][], error out=w271:errorcluster)
        n136 = Empty Array?(array=w272) -> (empty?=w273:bool)
        n137 = case shown="True" w273 {
          tunnel: [w289 w297] -> w260
          tunnel: w271 -> [w287 w298]
          tunnel: w272 -> [w284 _]
          tunnel: w274 -> [_ w293]
          tunnel: w275 -> [_ w292]
          frame False {
            w282 = 0 ("index (row)")
            n138 = Index Array(array=w284, index (row) #2=w282, index (col) #2=w282, index (row) #3=w282, index (col) #3=1 ("disabled index (col)"), index (row) #4=w282, index (col) #4=2 ("disabled index (col)")) -> (element #2=w286:string, element #3=w279:string, element #4=w280:string)  [unwired: 2 in, 1 out]
            n139 = Decimal String To Number(string=w280) -> (number=w283:i32)  [unwired: 2 in, 1 out]
            n140 = call "FGV_REWORK_login.vi"("options"=FGV_REWORK_login."login", "error_in"=w287, "access_level_in"=w283, "username_in"=w279, "ID_in"=w286) -> ("error_out"=w289:errorcluster)  [unwired: 3 in, 3 out]
          }
          frame True {
            n141 = call-poly "Get Localized Phrase Compact Interface.vi"("Key"="Scanned card not in database!\nCard: %s\nHash: %s" ("Message")) -> ("Translated Phrase"=w290:string)
            n142 = Format Into String(format string=w290, w293, w292) -> (resulting string=w291:string)  [unwired: 2 in, 1 out]
            n143 = call "message_popup.vi"("Warning(T)/Info(F)"=TRUE, "error_in"=w298, "Message"=w291, "Title"="Login", "Button Label"="OK") -> ("error_out"=w297:errorcluster)  [unwired: 6 in]
          }
        }
        n144 = call "REWORK_MAIN_check_for_error.vi"("MAIN_loop_state_in"=REWORK_MAIN_sequence_state."get_next_state", "error_in"=w260) -> ("MAIN_loop_state_out"=w277:T9, "error_out"=w278:errorcluster)  [unwired: 8 in]
      }
      frame "USER_logout" {
        n145 = call "FGV_REWORK_login.vi"("options"=FGV_REWORK_login."logout", "error_in"=w301) -> ("error_out"=w300:errorcluster)  [unwired: 6 in, 3 out]
        n146 = call "REWORK_MAIN_check_for_error.vi"("MAIN_loop_state_in"=REWORK_MAIN_sequence_state."clear_gear_data", "error_in"=w300) -> ("MAIN_loop_state_out"=w304:T9, "error_out"=w305:errorcluster)  [unwired: 8 in]
      }
      frame "clear_gear_data" {
        n147 = call "FGV_REWORK_records_display.vi"("options"=FGV_REWORK_records_display."clear", "error_in"=w309) -> ("error_out"=w308:errorcluster)  [unwired: 8 in, 1 out]
        n148 = call "FGV_REWORK_status_display.vi"("options"=FGV_REWORK_status_display."clear", "error_in"=w308) -> ("error_out"=w307:errorcluster)  [unwired: 9 in]
        n149 = call "FGV_REWORK_destination_selector.vi"("options"=FGV_REWORK_destination_selector."clear", "error_in"=w307) -> ("error_out"=w306:errorcluster)  [unwired: 8 in, 1 out]
        n150 = local write "gear_serial_display"("") -> ()
        n151 = call "REWORK_MAIN_check_for_error.vi"("MAIN_loop_state_in"=REWORK_MAIN_sequence_state."get_next_state", "error_in"=w306) -> ("MAIN_loop_state_out"=w315:T9, "error_out"=w316:errorcluster)  [unwired: 8 in]
      }
      frame "error" {
        n152 = call <vilib>:"Clear Errors.vi"("error in (no error)"=w320) -> ("error out"=w322:errorcluster)  [unwired: 5 in, 1 out]
        n153 = call "FGV_REWORK_SQL_connection.vi"("options"=FGV_REWORK_SQL_connection."connection_active?", "error_in"=w322) -> ("error_out"=w323:errorcluster, "connection_active?"=w324:bool)  [unwired: 5 in, 3 out]
        n154 = case shown="False" w324 {
          tunnel: [w330 REWORK_MAIN_sequence_state."get_next_state" ("ST_TCP_sequence_state")] -> w318
          tunnel: [w329 w343] -> w319
          tunnel: w323 -> [w334 w343]
          tunnel: w317 -> [w327 _]
          frame False {
            # "ERROR WITH CONNECTION"
            n155 = Unbundle By Name(w327) -> ("queue_refnums.MAIN_queue"=w326:refnum<queue>)
            n156 = local write "SQL_connections_indicator_global"(TRUE ("SQL_connections_indicator_global")) -> ()
            n157 = To Variant(anything=PLC_connection_status."Error") -> (Variant=w337:variant)
            n158 = call "FGV_REWORK_DIAGNOSTICS_records_display.vi"("options"=FGV_REWORK_DIAGNOSTICS_records_display."set_SQL_connection_status", "error_in"=w334, "input"=w337) -> ("error_out"=w333:errorcluster)  [unwired: 7 in, 1 out]
            n159 = call "FGV_REWORK_SQL_connection.vi"("options"=FGV_REWORK_SQL_connection."disconnect", "error_in"=w333) -> ("error_out"=w340:errorcluster)  [unwired: 5 in, 4 out]
            n160 = call <vilib>:"Clear Errors.vi"("error in (no error)"=w340) -> ("error out"=w328:errorcluster)  [unwired: 5 in, 1 out]
            n161 = Preview Queue Element(queue=w326, timeout in ms (-1)=0, error in (no error)=w328) -> (element=w325:T22, error out=w329:errorcluster)  [unwired: 2 out]
            n162 = Unbundle By Name(w325) -> ("state"=w332:T9)
            n163 = case shown="Default" w332 {
              tunnel: [REWORK_MAIN_sequence_state."initialize" ("state") REWORK_MAIN_sequence_state."stop" ("state")] -> w330
              frame Default {
              }
              frame "stop" {
              }
            }
          }
          frame True {
            # "ERROR WITH SQL STATEMENT OR SIMILAR"
          }
        }
        n164 = call "wait_on_initialization.vi"("state"=w318) -> ()  [unwired: 11 in]
      }
      frame "stop" {
      }
    }
  }
  n165 = while {
    tunnel: w20 -> [w352]
    shift-right: [w356] -> _
    shift-left: _ -> [w354]
    shift-right: [w355] -> _
    shift-left: _ -> [w353]
    shift-right: [w350] -> w47
    shift-left: w71 -> [w351]
    shift-right: [w349] -> _
    shift-left: REWORK_TCP_sequence_state."initialize" ("PLC_TCP_loop_state_in") -> [w348]
    stop <- w357 stop-if-true
    # "TCP LISTENER"
    n166 = case shown="\"wait_for_connection\"" w348 {
      tunnel: [_ _ _ _ TRUE] -> w357
      tunnel: w351 -> [w358 w372 w403 w422 w428]
      tunnel: [w365 w384 w402 w425 w426] -> w350
      tunnel: [w369 w381 w406 w421 w427] -> w356
      tunnel: w354 -> [_ w381 w406 w421 _]
      tunnel: w352 -> [w361 _ w391 _ _]
      tunnel: [w364 w382 w401 w423 REWORK_TCP_sequence_state."stop" ("PLC_TCP_loop_state_in")] -> w349
      tunnel: [refnum<k5> refnum ("connection ID") w380 w396 w420 w427] -> w355
      tunnel: w353 -> [_ _ w396 w420 _]
      frame "initialize" {
        n167 = Unbundle By Name(w361) -> ("main_ini_file.ST 140 listener IP"=w360:string, "main_ini_file.ST 140 listener port"=w359:u16)
        n168 = String To IP(1:w360) -> (0:w368:u32)
        n169 = TCP Create Listener(7:w368, 8:w358, 10:w359) -> (0:w367:errorcluster, 3:w369:refnum<k5>)  [unwired: 2 in, 1 out]
        n170 = call "FGV_REWORK_connection_reference.vi"("options"=FGV_REWORK_connection_reference."set_listener_ID", "error_in"=w367, "reference_in"=w369) -> ("error_out"=w366:errorcluster)  [unwired: 5 in, 3 out]
        n171 = call "REWORK_TCP_check_for_error.vi"("PLC_TCP_loop_state_in"=REWORK_TCP_sequence_state."wait_for_connection", "error_in"=w366) -> ("PLC_TCP_loop_state_out"=w364:T15, "error_out"=w365:errorcluster)  [unwired: 8 in]
      }
      frame "wait_for_connection" {
        n172 = To Variant(anything=PLC_connection_status."Waiting" ("connection_status")) -> (Variant=w373:variant)
        n173 = call "FGV_REWORK_DIAGNOSTICS_records_display.vi"("options"=FGV_REWORK_DIAGNOSTICS_records_display."set_PLC_connection_status", "error_in"=w372, "input"=w373) -> ("error_out"=w371:errorcluster)  [unwired: 7 in, 1 out]
        n174 = TCP Wait On Listener(8:w371, 10:FALSE ("resolve remote address (T)"), 11:w381) -> (0:w378:errorcluster, 1:w376:u16, 2:w377:string, 4:w380:refnum<k5>)  [unwired: 1 in, 1 out]
        n175 = call "REWORK_set_IP_and_port_after_connection_established.vi"("error_in"=w378, "PLC_port"=w376, "PLC_IP"=w377) -> ("error_out"=w379:errorcluster)  [unwired: 8 in]
        n176 = call "FGV_REWORK_connection_reference.vi"("options"=FGV_REWORK_connection_reference."set_connection_ID", "error_in"=w379, "reference_in"=w380) -> ("error_out"=w385:errorcluster)  [unwired: 5 in, 3 out]
        n177 = call "REWORK_TCP_check_for_error.vi"("PLC_TCP_loop_state_in"=REWORK_TCP_sequence_state."handle_message" ("PLC_TCP_1_loop_states"), "error_in"=w385) -> ("PLC_TCP_loop_state_out"=w382:T15, "error_out"=w384:errorcluster)  [unwired: 8 in]
      }
      frame "handle_message" {
        n178 = Unbundle By Name(w391) -> ("queue_refnums.MAIN_queue"=w390:refnum<queue>)
        n179 = TCP Read(connection ID=w396, bytes to read=9999, error in (no error)=w403, 7:T23."Immediate" ("mode (standard)"), 9:-1 ("timeout ms (25000)")) -> (data out=w392:string, error out=w398:errorcluster)  [unwired: 1 out]
        n180 = To Variant(anything=w392) -> (Variant=w397:variant)
        n181 = Bundle By Name(cluster=T22 {"state"=enum."initialize", "variable"=variant} ("MANUAL_SQL_CON_queue_element"), "state"=REWORK_MAIN_sequence_state."parse_TCP", "variable"=w397) -> (w399:T22)
        n182 = Enqueue Element(queue=w390, element=w399, error in (no error)=w398) -> (error out=w394:errorcluster)  [unwired: 1 in, 2 out]
        n183 = case shown="No Error" w394 {
          selector: w394 -> [w410 w412]
          tunnel: [w409 w412] -> w393
          tunnel: w392 -> [w408 _]
          frame No Error {
            n184 = To Variant(anything=w408) -> (Variant=w407:variant)
            n185 = call "FGV_REWORK_DIAGNOSTICS_message_history_buffer.vi"("options"=FGV_REWORK_DIAGNOSTICS_message_history_buffer."add_TCP_PLC_to_PC", "error_in"=w410, "input"=w407) -> ("error_out"=w409:errorcluster)  [unwired: 7 in, 1 out]
          }
          frame Error {
          }
        }
        n186 = call "REWORK_TCP_check_for_error.vi"("PLC_TCP_loop_state_in"=REWORK_TCP_sequence_state."handle_message", "error_in"=w393) -> ("PLC_TCP_loop_state_out"=w401:T15, "error_out"=w402:errorcluster)  [unwired: 8 in]
      }
      frame "error" {
        # "don't go to initialize, because listener should be created only once\nmaybe move it before loop later, don't know yet"
        n187 = call "FGV_REWORK_error_buffer.vi"("thread"=REWORK_thread."TCP", "option"=FGV_REWORK_error_buffer."display", "error_in"=w422) -> ("error_out"=w416:errorcluster)  [unwired: 7 in, 1 out]
        n188 = To Variant(anything=PLC_connection_status."Error" ("connection_status")) -> (Variant=w417:variant)
        n189 = call "FGV_REWORK_DIAGNOSTICS_records_display.vi"("options"=FGV_REWORK_DIAGNOSTICS_records_display."set_PLC_connection_status", "error_in"=w416, "input"=w417) -> ("error_out"=w415:errorcluster)  [unwired: 7 in, 1 out]
        n190 = call "REWORK_TCP_check_for_error.vi"("PLC_TCP_loop_state_in"=REWORK_TCP_sequence_state."wait_for_connection", "error_in"=w415) -> ("PLC_TCP_loop_state_out"=w423:T15, "error_out"=w425:errorcluster)  [unwired: 8 in]
        n191 = call "wait_on_initialization.vi"("state"=w423) -> ()  [unwired: 11 in]
      }
      frame "stop" {
        w427 = refnum<k5> refnum ("connection ID")
        n192 = call <vilib>:"Clear Errors.vi"("error in (no error)"=w428) -> ("error out"=w426:errorcluster)  [unwired: 5 in, 1 out]
      }
    }
  }
  n193 = while {
    tunnel: w20 -> [w434]
    shift-right: [w440] -> _
    shift-left: "" -> [w437]
    shift-right: [w441] -> _
    shift-left: FALSE -> [w438]
    shift-right: [w442] -> _
    shift-left: _ -> [w439]
    shift-right: [w432] -> _
    shift-left: REWORK_SCANNER_sequence_state."initialize" ("REWORK_SCANNER_sequence_state") -> [w433]
    shift-right: [w431] -> w46
    shift-left: w71 -> [w435]
    stop <- w436 stop-if-true
    # "SCANNER"
    n194 = case shown="\"initialize\"" w433 {
      tunnel: w435 -> [w459 w475 w505 w542 w558 w568]
      tunnel: [w462 w473 w508 w543 w549 w566] -> w431
      tunnel: [w460 w468 w506 w541 w548 REWORK_SCANNER_sequence_state."stop" ("state")] -> w432
      tunnel: [_ _ _ _ _ TRUE] -> w436
      tunnel: w434 -> [w457 w474 w498 _ w552 _]
      tunnel: [w446 w464 w504 w545 w559 refnum<visa-resource-name> refnum ("VISA resource name out")] -> w442
      tunnel: w439 -> [_ w464 w504 w545 w559 w565]
      tunnel: w438 -> [_ w472 _ _ _ _]
      tunnel: [FALSE w472 w499 FALSE FALSE FALSE] -> w441
      tunnel: w437 -> [_ w470 w494 _ _ _]
      tunnel: ["" w470 w496 "" "" ""] -> w440
      frame "initialize" {
        n195 = Unbundle By Name(w457) -> ("main_ini_file.SCANNER Termination char"=w447:u8, "main_ini_file.SCANNER COM port"=w456:u16, "main_ini_file.SCANNER Baud rate"=w452:u32, "main_ini_file.SCANNER Data bits"=w451:u16, "main_ini_file.SCANNER Pairity"=w450:enum16{"None", "Odd", "Even", "Mark", "Space"}, "main_ini_file.SCANNER Stop bits"=w449:u16, "main_ini_file.SCANNER Flow control"=w448:u16)
        n196 = Number To Decimal String(number=w456) -> (decimal integer string=w455:string)  [unwired: 1 in]
        n197 = Concatenate Strings("COM" ("string"), w455) -> (w453:string)
        n198 = call-poly "VISA Configure Serial Port"("VISA resource name"=w453, "timeout (10sec)"=u32 150, "termination char\n(0xA = '\\n' = LF)"=w447, "baud rate (9600)"=w452, "data bits (8)"=w451, "parity (0:none)"=w450, "error in (no error)"=w459, "stop bits (10: 1 bit)"=w449, "flow control (0:none)"=w448) -> ("VISA resource name out"=w446:refnum<visa-resource-name>, "error out"=w458:errorcluster)  [unwired: 1 in, 4 out]
        n199 = call "REWORK_SCANNER_check_for_error.vi"("SCANNER_loop_state_in"=REWORK_SCANNER_sequence_state."get_next_state" ("SQL_EDITOR_sequence_state"), "error_in"=w458) -> ("SCANNER_loop_state_out"=w460:T17, "error_out"=w462:errorcluster)  [unwired: 8 in]
      }
      frame "get_next_state" {
        n200 = Unbundle By Name(w474) -> ("queue_refnums.SCANNER_queue"=w476:refnum<queue>)
        n201 = case shown="True" w472 {
          tunnel: [-1 ("timeout in ms (-1)") 0 ("timeout in ms (-1)")] -> w471
          frame False {
          }
          frame True {
          }
        }
        n202 = Dequeue Element(queue=w476, timeout in ms (-1)=w471, error in (no error)=w475) -> (element=w463:T25, timed out?=w465:bool, error out=w467:errorcluster)  [unwired: 1 out]
        n203 = case shown="False" w465 {
          tunnel: w463 -> [w477 _]
          tunnel: [w478 REWORK_SCANNER_sequence_state."read" ("REWORK_SCANNER_sequence_state")] -> w469
          tunnel: [w481 w490] -> w466
          tunnel: w467 -> [w482 w490]
          tunnel: w464 -> [w480 _]
          frame False {
            # "clear buffers\non read start"
            n204 = Unbundle By Name(w477) -> ("state"=w479:T17)
            n205 = case shown="\"read\"" w479 {
              selector: w479 -> [w484 w485]
              tunnel: w482 -> [w483 w488]
              tunnel: [w483 w487] -> w481
              tunnel: w480 -> [_ w486]
              tunnel: [w484 w485] -> w478
              frame Default {
              }
              frame "read" {
                n206 = VISA Clear(VISA resource name=w486, error in (no error)=w488) -> (error out=w487:errorcluster)  [unwired: 1 out]
              }
            }
          }
          frame True {
          }
        }
        n207 = call "REWORK_SCANNER_check_for_error.vi"("SCANNER_loop_state_in"=w469, "error_in"=w466) -> ("SCANNER_loop_state_out"=w468:T17, "error_out"=w473:errorcluster)  [unwired: 8 in]
      }
      frame "read" {
        # "timeout"
        n208 = VISA Read(VISA resource name=w504, byte count=u32 9999, error in (no error)=w505) -> (read buffer=w497:string, return count=w500:u32, error out=w495:errorcluster)  [unwired: 1 out]
        n209 = case shown="No Error" w495 {
          tunnel: w500 -> [_ w532]
          tunnel: [w517 w531] -> w499
          tunnel: w498 -> [w516 w530]
          tunnel: w497 -> [w511 w529]
          tunnel: [w515 w528] -> w496
          tunnel: w494 -> [w512 w527]
          tunnel: TRUE -> [w514 w526]
          frame No Error {
            # "no (timeout) error means that termination character was encountered"
            n210 = Concatenate Strings(w512, w511) -> (w510:string)
            n211 = Not Equal?(x=w510, y="NoRead\r\n" ("x")) -> (x != y?=w509:bool)
            n212 = case shown="True" w509 {
              tunnel: [FALSE w525] -> w517
              tunnel: w516 -> [w522 _]
              tunnel: ["" ""] -> w515
              tunnel: w514 -> [_ w525]
              tunnel: w510 -> [w518 _]
              frame True {
                # "read successful - send data and stop reading"
                n213 = call <vilib>:"Trim Whitespace.vi"("string"=w518) -> ("trimmed string"=w519:string)  [unwired: 1 in]
                n214 = Unbundle By Name(w522) -> ("queue_refnums.SCANNER_data"=w521:refnum<queue>)
                n215 = Lossy Enqueue Element(queue=w521, element=w519) -> ()  [unwired: 1 in, 4 out]
              }
              frame False {
                # "read completed, but unsuccessful - clear buffer and start read again"
              }
            }
          }
          frame Error {
            # "(timeout) error and some bytes read means that timeout occured before encountering termination character"
            n216 = case shown="0" w532 {
              tunnel: [w536 w537] -> w531
              tunnel: w530 -> [_ _]
              tunnel: w529 -> [w534 _]
              tunnel: [w533 w538] -> w528
              tunnel: w527 -> [w535 w538]
              tunnel: w526 -> [w536 w537]
              frame Default {
                # "if error and some bytes read, append new bytes (probably timeout, if not error case will take care of it)"
                n217 = Concatenate Strings(w535, w534) -> (w533:string)
              }
              frame 0 {
                # "if error and no bytes read, do nothing (probably timeout, if not error case will take care of it)"
                # "if error and no bytes read, do nothing (probably timeout, if not error case takes care of it"
              }
            }
          }
        }
        n218 = call <vilib>:"Clear Errors.vi"("error in (no error)"=w495, "specific error code to clear (0: all)"=-1073807339) -> ("error out"=w502:errorcluster)  [unwired: 4 in, 1 out]
        n219 = call "REWORK_SCANNER_check_for_error.vi"("SCANNER_loop_state_in"=REWORK_SCANNER_sequence_state."get_next_state" ("state"), "error_in"=w502) -> ("SCANNER_loop_state_out"=w506:T17, "error_out"=w508:errorcluster)  [unwired: 8 in]
      }
      frame "cancel_read" {
        n220 = call "REWORK_SCANNER_check_for_error.vi"("SCANNER_loop_state_in"=REWORK_SCANNER_sequence_state."get_next_state", "error_in"=w542) -> ("SCANNER_loop_state_out"=w541:T17, "error_out"=w543:errorcluster)  [unwired: 8 in]
      }
      frame "error" {
        n221 = Unbundle By Name(w552) -> ("queue_refnums.SCANNER_queue"=w551:refnum<queue>)
        n222 = call "FGV_REWORK_error_buffer.vi"("thread"=REWORK_thread."SCANNER", "option"=FGV_REWORK_error_buffer."display", "error_in"=w558) -> ("error_out"=w550:errorcluster)  [unwired: 7 in, 1 out]
        n223 = Preview Queue Element(queue=w551, timeout in ms (-1)=0, error in (no error)=w550) -> (element=w555:T25, error out=w549:errorcluster)  [unwired: 2 out]
        n224 = Unbundle By Name(w555) -> ("state"=w553:T17)
        n225 = case shown="\"stop\"" w553 {
          tunnel: [REWORK_SCANNER_sequence_state."initialize" ("state") REWORK_SCANNER_sequence_state."stop" ("state")] -> w548
          frame Default {
          }
          frame "stop" {
          }
        }
        n226 = call "wait_on_initialization.vi"("state"=w548) -> ()  [unwired: 11 in]
      }
      frame "stop" {
        # "1. takes so long to close it\nmaybe its not needed?\n2. works faster on server and is needed\nerrors after restart if not closed properly"
        n227 = call <vilib>:"Clear Errors.vi"("error in (no error)"=w568) -> ("error out"=w567:errorcluster)  [unwired: 5 in, 1 out]
        n228 = VISA Close(VISA resource name=w565, error in (no error)=w567) -> (error out=w566:errorcluster)
      }
    }
  }
  n229 = while {
    tunnel: w71 -> [w575]
    tunnel: [w574] -> w49
    tunnel: w20 -> [w572]
    tunnel: w19 -> [w571]
    stop <- w573 stop-if-true
    # "EVENTS"
    n230 = event shown="[15] Menu Selection (User)" {
      selector: _ -> [_ _ _ _ _ _ _ _ _ _ _ _ _ _ _ _ _]
      dyn-events: _ -> [_ _ _ _ _ _ _ _ _ _ _ _ _ _ _ _ _]
      timeout: w571 -> [_ _ _ _ _ _ _ _ _ _ _ _ _ _ _ _ _]
      tunnel: w575 -> [w577 w579 w582 w584 w587 w600 w602 w608 w628 w631 w638 w663 w667 w703 w726 w734 w753]
      tunnel: [w576 w578 w581 w584 w586 w599 w603 w607 w621 w630 w637 w663 w670 w702 w726 w734 w753] -> w574
      tunnel: [_ _ _ _ _ _ _ _ _ _ _ _ w669 _ _ _ _] -> w573
      tunnel: w572 -> [_ _ _ _ w585 w598 w601 w606 _ _ _ _ w671 w701 _ _ _]
      event "DIAGNOSTICS_records": Double Click {
        n231 = event-data() -> ()  [unwired: 1 in, 9 out]
        n232 = call "REWORK_display_messages_history.vi"("error_in"=w577) -> ("error_out"=w576:errorcluster)  [unwired: 10 in]
      }
      event "DIAGNOSTICS_save_log": Value Change {
        n233 = event-data() -> ()  [unwired: 1 in, 6 out]
        n234 = call "FGV_REWORK_DIAGNOSTICS_message_history_buffer.vi"("options"=FGV_REWORK_DIAGNOSTICS_message_history_buffer."save_log", "error_in"=w579) -> ("error_out"=w578:errorcluster)  [unwired: 8 in, 1 out]
      }
      event "DIAGNOSTICS_show_messages": Value Change {
        n235 = event-data() -> ()  [unwired: 1 in, 6 out]
        n236 = call "REWORK_display_messages_history.vi"("error_in"=w582) -> ("error_out"=w581:errorcluster)  [unwired: 10 in]
      }
      event "ERROR_clear": Value Change {
        n237 = event-data() -> ()  [unwired: 1 in, 6 out]
        n238 = call "FGV_REWORK_error_buffer.vi"("option"=FGV_REWORK_error_buffer."clear") -> ()  [unwired: 9 in, 2 out]
      }
      event "REWORK_commit": Value Change {
        n239 = event-data() -> ()  [unwired: 1 in, 1 out]
        n240 = Unbundle By Name(w585) -> ("queue_refnums.MAIN_queue"=w589:refnum<queue>)
        n241 = Enqueue Element(queue=w589, element=T22 {"state"=enum."REWORK_commit", "variable"=variant}, error in (no error)=w587) -> (error out=w586:errorcluster)  [unwired: 1 in, 2 out]
      }
      event "REWORK_read_data": Value Change {
        # "THIS IS FAKE TCP TO EASILY REUSE CODE FOR TCP MESSAGE PARSING\nHOPE IT WOULD NOT BITE\ncommand is 101 instead of 1"
        n242 = event-data() -> ()  [unwired: 1 in, 6 out]
        n243 = local read "REWORK_gear_serial"() -> (w590:string)
        n244 = Byte Array To String(unsigned byte array=u8[] [101, 255, 255]) -> (string=w593:string)
        n245 = Concatenate Strings(w593, w590) -> (w591:string)
        n246 = Unbundle By Name(w598) -> ("queue_refnums.MAIN_queue"=w597:refnum<queue>)
        n247 = To Variant(anything=w591) -> (Variant=w592:variant)
        n248 = Bundle By Name(cluster=T22 {"state"=enum."parse_TCP", "variable"=variant} ("element"), "variable"=w592) -> (w595:T22)
        n249 = Enqueue Element(queue=w597, element=w595, error in (no error)=w600) -> (error out=w599:errorcluster)  [unwired: 1 in, 2 out]
      }
      event "REWORK_clear_gear_data": Value Change {
        n250 = event-data() -> ()  [unwired: 1 in, 6 out]
        n251 = Unbundle By Name(w601) -> ("queue_refnums.MAIN_queue"=w605:refnum<queue>)
        n252 = Enqueue Element(queue=w605, element=T22 {"state"=enum."clear_gear_data", "variable"=variant}, error in (no error)=w602) -> (error out=w603:errorcluster)  [unwired: 1 in, 2 out]
      }
      event Timeout {
        n253 = event-data() -> ()  [unwired: 1 in, 3 out]
        n254 = local read "current_access_level"() -> (w609:i32)
        n255 = case shown="Default" w609 {
          tunnel: w608 -> [w610 w611]
          tunnel: [w610 w619] -> w607
          tunnel: w606 -> [_ w613]
          frame 0 {
          }
          frame Default {
            n256 = Unbundle By Name(w613) -> ("queue_refnums.MAIN_queue"=w615:refnum<queue>)
            n257 = Enqueue Element(queue=w615, element=T22 {"state"=enum."USER_logout", "variable"=variant}, error in (no error)=w611) -> (error out=w612:errorcluster)  [unwired: 1 in, 2 out]
            n258 = call "message_popup.vi"("Warning(T)/Info(F)"=TRUE, "error_in"=w612, "Message"="Automatic user logout was performed due to inactivity", "Title"="Automatic Logout", "Button Label"="OK") -> ("error_out"=w619:errorcluster)  [unwired: 6 in]
          }
        }
      }
      event "REWORK_records": Double Click {
        n259 = event-data() -> ("Row"=w626:i32)  [unwired: 1 in]
        n260 = To Variant(anything=w626) -> (Variant=w627:variant)
        n261 = call "FGV_REWORK_records_display.vi"("options"=FGV_REWORK_records_display."toggle_results", "error_in"=w628, "input"=w627) -> ("error_out"=w622:errorcluster)  [unwired: 7 in, 1 out]
        n262 = local read "REWORK_station_filter"() -> (w625:T1)
        n263 = To Variant(anything=w625) -> (Variant=w624:variant)
        n264 = call "FGV_REWORK_records_display.vi"("options"=FGV_REWORK_records_display."display", "error_in"=w622, "input"=w624) -> ("error_out"=w621:errorcluster)  [unwired: 7 in, 1 out]
      }
      event Value Change {
        n265 = event-data() -> ("NewVal"=w632:T1)  [unwired: 1 in, 5 out]
        n266 = To Variant(anything=w632) -> (Variant=w634:variant)
        n267 = call "FGV_REWORK_records_display.vi"("options"=FGV_REWORK_records_display."display", "error_in"=w631, "input"=w634) -> ("error_out"=w630:errorcluster)  [unwired: 7 in, 1 out]
      }
      event "REWORK_toggle_all_results": Value Change {
        n268 = event-data() -> ()  [unwired: 1 in, 1 out]
        n269 = local read "REWORK_toggle_all_results"() -> (w636:bool)
        n270 = case shown="False" w636 {
          selector: w636 -> [w643 w655]
          tunnel: [w647 w659] -> w637
          tunnel: w638 -> [w650 w662]
          tunnel: [w642 w654] -> w635
          frame True {
            n271 = call "FGV_REWORK_records_display.vi"("options"=FGV_REWORK_records_display."hide_all_results", "error_in"=w650) -> ("error_out"=w648:errorcluster)  [unwired: 8 in, 1 out]
            n272 = call-poly "Get Localized Phrase Compact Interface.vi"("Key"="SHOW ALL RESULTS" ("Boolean Text.Text")) -> ("Translated Phrase"=w639:string)
            n273 = property on="REWORK_toggle_all_results" class="Bool"("BoolText.Text"=w639) -> ()  [unwired: 2 in, 2 out]
            n274 = local read "REWORK_station_filter"() -> (w645:T1)
            n275 = To Variant(anything=w645) -> (Variant=w644:variant)
            n276 = property on="REWORK_records" class="MCListbox (strict)"("TopLeft"=T26 {"Row"=0, "Column"=0} ("Active Cell:Active Cell")) -> ()  [unwired: 2 in, 2 out]
            n277 = call "FGV_REWORK_records_display.vi"("options"=FGV_REWORK_records_display."display", "error_in"=w648, "input"=w644) -> ("error_out"=w647:errorcluster)  [unwired: 7 in, 1 out]
            n278 = Not(x=w643) -> (.not. x?=w642:bool)
          }
          frame False {
            n279 = call "FGV_REWORK_records_display.vi"("options"=FGV_REWORK_records_display."show_all_results", "error_in"=w662) -> ("error_out"=w660:errorcluster)  [unwired: 8 in, 1 out]
            n280 = call-poly "Get Localized Phrase Compact Interface.vi"("Key"="HIDE ALL RESULTS" ("Boolean Text.Text")) -> ("Translated Phrase"=w651:string)
            n281 = property on="REWORK_toggle_all_results" class="Bool"("BoolText.Text"=w651) -> ()  [unwired: 2 in, 2 out]
            n282 = local read "REWORK_station_filter"() -> (w657:T1)
            n283 = To Variant(anything=w657) -> (Variant=w656:variant)
            n284 = property on="REWORK_records" class="MCListbox (strict)"("TopLeft"=T26 {"Row"=0, "Column"=0} ("Active Cell:Active Cell")) -> ()  [unwired: 2 in, 2 out]
            n285 = call "FGV_REWORK_records_display.vi"("options"=FGV_REWORK_records_display."display", "error_in"=w660, "input"=w656) -> ("error_out"=w659:errorcluster)  [unwired: 7 in, 1 out]
            n286 = Not(x=w655) -> (.not. x?=w654:bool)
          }
        }
        n287 = local write "REWORK_toggle_all_results"(w635) -> ()
      }
      event "REWORK_destination": Mouse Down? {
        n288 = event-data() -> ()  [unwired: 1 in, 8 out]
        n289 = call "FGV_REWORK_destination_selector.vi"("options"=FGV_REWORK_destination_selector."display_values") -> ()  [unwired: 9 in, 2 out]
        n290 = event-data("Discard?"=FALSE) -> ()  [unwired: 4 in, 1 out]
      }
      event "STOP": Value Change {
        n291 = event-data() -> ()  [unwired: 1 in, 6 out]
        n292 = disable-structure shown="RUN_TIME_ENGINE==True" {
          disable-tunnel: [w674 TRUE ("Result")] -> w668
          disable-tunnel: w667 -> [w673 w685]
          disable-tunnel: [w672 w685] -> w666
          frame condition #0 {
            n293 = case shown="No Error" w673 {
              selector: w673 -> [w679 w683]
              tunnel: [w680 TRUE ("Result")] -> w674
              tunnel: [w678 w683] -> w672
              frame No Error {
                n294 = call "confirm_popup.vi"("Warning(T)/Inf(F)"=TRUE, "error_in"=w679, "False Label"="No", "True Label"="Yes", "Message"="Are you sure you want to exit the application?") -> ("error_out"=w678:errorcluster, "Result"=w680:bool)  [unwired: 5 in]
              }
              frame Error {
              }
            }
          }
          frame condition #1 (active) {
          }
        }
        n295 = case shown="True" w668 {
          tunnel: w666 -> [w687 w700]
          tunnel: w671 -> [_ w698]
          tunnel: [w687 w694] -> w670
          tunnel: [FALSE TRUE] -> w669
          frame False {
          }
          frame True {
            n296 = Unbundle By Name(w698) -> ("queue_refnums.SCANNER_queue"=w699:refnum<queue>, "queue_refnums.MAIN_queue"=w691:refnum<queue>)
            n297 = call <vilib>:"Clear Errors.vi"("error in (no error)"=w700) -> ("error out"=w693:errorcluster)  [unwired: 5 in, 1 out]
            n298 = Enqueue Element At Opposite End(queue=w691, element=T22 {"state"=enum."stop", "variable"=variant}, error in (no error)=w693) -> (error out=w692:errorcluster)  [unwired: 1 in, 2 out]
            n299 = Enqueue Element At Opposite End(queue=w699, element=T25 {"state"=enum."stop", "variable"=variant}, error in (no error)=w692) -> (error out=w696:errorcluster)  [unwired: 1 in, 2 out]
            n300 = call "FGV_REWORK_DIAGNOSTICS_message_history_buffer.vi"("options"=FGV_REWORK_DIAGNOSTICS_message_history_buffer."save_log", "error_in"=w696) -> ("error_out"=w694:errorcluster)  [unwired: 8 in, 1 out]
            n301 = call "FGV_REWORK_connection_reference.vi"("options"=FGV_REWORK_connection_reference."KILL_ALL_CONNECTIONS") -> ()  [unwired: 7 in, 4 out]
          }
        }
      }
      event "USER_login_logout": Value Change {
        n302 = event-data() -> ()  [unwired: 1 in, 6 out]
        n303 = local read "current_access_level"() -> (w704:i32)
        n304 = case shown="0" w704 {
          tunnel: [w710 w724] -> w702
          tunnel: w703 -> [w709 w722]
          tunnel: w701 -> [w708 w721]
          frame 0 {
            n305 = call "REWORK_LOGIN_scan_barcode.vi"("error_in"=w709, "all_config_info"=w708) -> ("error_out"=w707:errorcluster, "Canceled?"=w705:bool, "barcode"=w706:string)  [unwired: 7 in]
            n306 = case shown="True" w705 {
              tunnel: [w718 w719] -> w710
              tunnel: w707 -> [w715 w719]
              tunnel: w708 -> [w714 _]
              tunnel: w706 -> [w713 _]
              frame False {
                n307 = Unbundle By Name(w714) -> ("queue_refnums.MAIN_queue"=w717:refnum<queue>)
                n308 = To Variant(anything=w713) -> (Variant=w716:variant)
                n309 = Bundle By Name(cluster=T22 {"state"=enum."USER_login", "variable"=variant} ("element"), "variable"=w716) -> (w711:T22)
                n310 = Enqueue Element(queue=w717, element=w711, error in (no error)=w715) -> (error out=w718:errorcluster)  [unwired: 1 in, 2 out]
              }
              frame True {
              }
            }
          }
          frame Default {
            n311 = Unbundle By Name(w721) -> ("queue_refnums.MAIN_queue"=w723:refnum<queue>)
            n312 = Enqueue Element(queue=w723, element=T22 {"state"=enum."USER_logout", "variable"=variant}, error in (no error)=w722) -> (error out=w724:errorcluster)  [unwired: 1 in, 2 out]
          }
        }
      }
      event "current_access_level": Value Change {
        n313 = event-data() -> ("NewVal"=w728:i32)  [unwired: 1 in]
        n314 = case shown="1..10" w728 {
          tunnel: [w730 w731] -> w727
          frame Default {
            w730 = enum32{"Rework", "Diagnostics", "Errors"}[] [enum."Errors"] items=["Rework", "Diagnostics", "Errors"]
          }
          frame 1..10 {
            w731 = enum32{"Rework", "Diagnostics", "Errors"}[] [enum."Rework", enum."Diagnostics", enum."Errors"] items=["Rework", "Diagnostics", "Errors"]
          }
        }
        n315 = control-ref of="main_tab"() -> (w725:refnum<vi>)
        n316 = control-ref of="This VI"() -> (w729:refnum<vi>)
        n317 = call "REWORK_show_hide_pages.vi"("This VI"=w729, "visible_pages"=w727, "main_tab_ref"=w725) -> ()  [unwired: 9 in]
      }
      event Menu Selection (User) {
        n318 = event-data() -> ("ItemTag"=w733:string)  [unwired: 1 in, 6 out]
        n319 = call "Get Key For Phrase.vi"("Phrase"=w733) -> ("Key"=w732:string)  [unwired: 9 in, 1 out]
        n320 = case shown="\"Language - English\", \"Language - Russian\"" w732 {
          selector: w732 -> [_ _ w749 _]
          frame Default {
          }
          frame "About" {
            n321 = call "Get Localized Phrase Compact Interface 0D.vi"("Key"="SQL Proxy Application\nMSG Assembly Line\nA603A00\n\nAumatic sp. z o.o.\nPilsudskiego 22\n32-050 Skawina\nPOLAND\n\nCOMPILATION DATE: %s\nCOMPILATION TIME: %s\nJakub Longa, 2020\n\n+48 (12) 256-77-90\naumatic.com" ("about_string")) -> ("Translated Phrase"=w735:string)
            n322 = disable-structure shown="Default" {
              disable-tunnel: [w741 w744] -> w738
              disable-tunnel: [w742 w744] -> w737
              frame condition #0 {
                n323 = vi-ref "get_exe_compilation_date.vi"() -> (w743:refnum<vi>)
                n324 = call-by-ref "?"(reference=w743) -> ("compilation_time"=w741:string, "compilation_date"=w742:string)  [unwired: 10 in, 3 out]
              }
              frame condition #1 (active) {
                n325 = call-poly "Get Localized Phrase Compact Interface.vi"("Key"="NOT COMPILED!" ("compilation_date")) -> ("Translated Phrase"=w744:string)
              }
            }
            n326 = Format Into String(format string=w735, w737, w738) -> (resulting string=w740:string)  [unwired: 2 in, 1 out]
            n327 = call "about_window.vi"("lines_to_bold"=i32[] [0, 1, 4, 9], "about_string"=w740) -> ()  [unwired: 9 in, 1 out]
          }
          frame "Language - English", "Language - Russian" {
            n328 = case shown="\"Language - English\", Default" w749 {
              tunnel: ["Russian" ("Target Language (current lang)") "English" ("Target Language (current lang)")] -> w748
              frame "Language - Russian" {
              }
              frame "Language - English", Default {
              }
            }
            n329 = call "Set Language.vi"("Target Language (current lang)"=w748) -> ("error out"=w746:errorcluster)  [unwired: 9 in, 1 out]
            n330 = Current VI's Menubar() -> (w747:refnum<k9>)
            n331 = call "REWORK_create_menu_bar.vi"("error_in"=w746, "menu_bar_refnum"=w747) -> ()  [unwired: 9 in, 1 out]
          }
          frame "Exit" {
            n332 = property on="STOP" class="Bool (strict)"("Val(Sgnl)"=TRUE ("Value (Signaling)")) -> ()  [unwired: 2 in, 2 out]
          }
        }
      }
      event Panel Close? {
        n333 = event-data() -> ()  [unwired: 1 in, 4 out]
        n334 = property on="STOP" class="Bool (strict)"("Val(Sgnl)"=TRUE ("Value (Signaling)")) -> ()  [unwired: 2 in, 2 out]
        n335 = event-data("Discard?"=TRUE) -> ()  [unwired: 1 in, 1 out]
      }
    }
  }
  n336 = Merge Errors(w49, w48, w47, w46) -> (w11:errorcluster)
  n337 = call "Uninitialize.vi"("error in"=w11) -> ("error out"=w10:errorcluster)  [unwired: 10 in]
  n338 = call "REWORK_destroy_queues.vi"("error_in"=w10, "all_config_info"=w20) -> ("error_out"=w72:errorcluster)  [unwired: 9 in]
  n339 = control-ref of="This VI"() -> (w74:refnum<vi>)
  n340 = call "close_front_panel_in_exe.vi"("error_in"=w72, "vi_reference_in"=w74) -> ("error_out"=w73:errorcluster)  [unwired: 9 in]
  n341 = call <vilib>:"Clear Errors.vi"("error in (no error)"=w73) -> ()  [unwired: 5 in, 2 out]
